vi "Actor Core.vi"(8 "error in":errorcluster, 11 "Rack Controller in":refnum<class "Rack Controller.lvclass">) -> (0 "error out":errorcluster, 3 "Actor out":refnum<class "Actor.lvclass">)   [LabVIEW 2019, in "Rack Controller.lvclass"]
doc: "(<B>Filename</B>: Actor Framework.lvlib:Actor.lvclass:Actor Core.vi)\n\nReceives messages to the actor, reacts to them, and initiates any error handling that may shut the actor down.\n\nDescendant classes may override this VI to append parallel tasks for the actor to complete while it handles messages. Overrides use the Call Parent Method node."
uses:
  Rack Controller.lvclass
  <vilib>/ActorFramework/Actor/Actor.lvclass
  <vilib>/ActorFramework/Stop Msg/Stop Msg.lvclass
  <vilib>/ActorFramework/Message Enqueuer/Message Enqueuer.lvclass
  Algorithm/FrameworkOverrides/Algorithm.lvclass
  <vilib>/vision/Image Controls.llb/IMAQ Image.ctl
  Controls/RC Local Data.ctl
  Controls/Output Cluster_RC.ctl
  Common/Controls/Camera Optics Diagnostics Result.ctl
  Common/Controls/Camera Optics Diagnostics.ctl
  Inspection Statemachine/Controls/Result Cluster_SM.ctl
  Inspection Statemachine/Inspection Statemachine.lvclass
  Controls/Part Details_RC.ctl
  Common/Controls/AllPartInfo.ctl
  <vilib>/event_ctls.llb/usereventprio.ctl
  ZenCAM/Camera Controller/Camera Controller Actor/Camera Controller.lvclass
  C:/Program Files/National Instruments/LabVIEW 2019/vi.lib/ActorFramework/Actor/Actor.lvclass
panel:
  out "Part Name":string
  out "RackId":i32
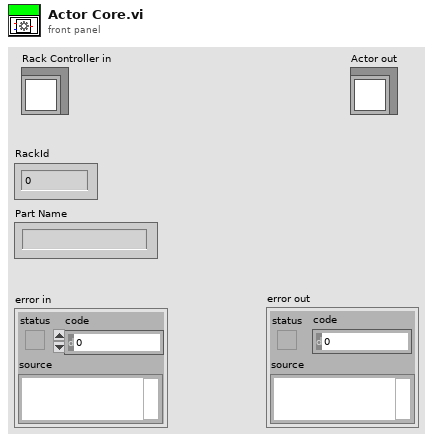
[diagram p1: front panel]
types:
  T1 = typedef "IMAQ Image.ctl" = refnum<image>
  T2 = cluster{"Buffer":cluster{"Result Cluster":cluster{"Rack ID":u8, "Measurement Values Array ":dbl[], "Images Array":T1[], "Result PF":bool, "Production Count Details":cluster{"Total Fail":u64, "Total Pass":u64, "Total Count":u64}, "Reel Count Details":cluster{"Reel Fail":u64, "Reel Pass":u64, "Reel Count":u64}, "Control PF Array":bool[], "Specification PF Array":bool[], "Specification Fail?":bool, "Reel Number":u64, "Status":string}, "Pause on Fail?":bool, "Total Count Finish?":bool, "Reel Count Finish?":bool}[], "Result Count":u32, "Swithch?":bool, "Check Pos 3":u32, "Global Count":u32, "Check Pos 1":u32, "Check Pos 2":u32, "Result ":cluster{"Result Cluster":cluster{"Rack ID":u8, "Measurement Values Array ":dbl[], "Images Array":T1[], "Result PF":bool, "Production Count Details":cluster{"Total Fail":u64, "Total Pass":u64, "Total Count":u64}, "Reel Count Details":cluster{"Reel Fail":u64, "Reel Pass":u64, "Reel Count":u64}, "Control PF Array":bool[], "Specification PF Array":bool[], "Specification Fail?":bool, "Reel Number":u64, "Status":string}, "Pause on Fail?":bool, "Total Count Finish?":bool, "Reel Count Finish?":bool}, "Image buffer":T1[][], "Buffer Size":u32}
  T3 = typedef "Rack Controller.lvclass/RC Local Data.ctl" = cluster{"Timeout":i32, "Core":cluster{"Current VI Reference":refnum<vi>, "Close Panel on Exit?":bool}, "Rack Id":u8, "Part Details":T4, "Ack":i32, "First Call?":bool, "Send Run to CC?":bool, "State":string, "Reel Number":u64, "Output Cluster":T5, "System Info_RC":cluster{"HardwareEmulated":bool, "DefectTrackingEnable":bool, "PauseOnReelCountFinish":bool, "StopOnTotalCountFinish":bool}, "Rack based Parameters":variant, "Update":bool, "CountDetails":cluster{"Total Cluster Values":cluster{"Total Fail":u64, "Total Pass":u64, "Total Count":u64}, "Reel Counter Cluster":cluster{"Reel Fail":u64, "Reel Pass":u64, "Reel Count":u64}}}
  T4 = typedef "Rack Controller.lvclass/Part Details_RC.ctl" = cluster{"Name":string, "Unload Position Counts":cluster{"Fail":u32, "Reel End":u32, "Production End":u32}, "Number Of Cameras":u8, "Measurement Details Array":cluster{"Measuement ID":u16, "Measurement Name":string, "Measurement Enable":bool, "CL Violation Threshold":cluster{"M":u8, "N":u64}, "SL Violation Threshold":cluster{"M":u8, "N":u64}, "CL Fail Count Array":u64[], "SL Fail Count Array":u64[]}[], "Reel Count":u64, "Total Count":u64}
  T5 = typedef "Rack Controller.lvclass/Output Cluster_RC.ctl" = cluster{"Acknowledgement":cluster{"Actor Enqueuer":refnum<class "Message Enqueuer.lvclass">, "VI Reference":refnum<vi>, "VI Name":string}, "Rack ID":u8, "Clear":bool, "Light Camera Info":T6, "Camera Optics Diagnostics Result":T7, "Receiver Enqueuer":cluster{"Actor Enqueuer":refnum<class "Message Enqueuer.lvclass">, "VI Name":string}, "Error Message":string, "Part Details":cluster{"Part Name":string, "Total Count":u64, "Reel Count":u64}, "Result Cluster":T8, "Part Info":cluster{"Part Name":string, "Rack ID":u8, "MeasurementIDsArray":u16[], "Measurement Names Array":string[], "Spec Values Array":cluster{"LCL":dbl, "UCL":dbl, "LSL":dbl, "USL":dbl, "Nominal Value":dbl}[], "Camera Names Array":string[], "Total count":u64, "Reel count":u64}, "AllPartInfo":T9, "ImagesAndCount":cluster{"Image Array":T1[], "ImageCount":u64}}
  T6 = typedef "Camera Optics Diagnostics.ctl" = cluster{"Light Camera Name":string, " State":string}
  T7 = typedef "Camera Optics Diagnostics Result.ctl" = cluster{"LightCameraName":string, "DiagnosedImage":T1, "DustPercentage":dbl, "Result":bool}
  T8 = typedef "Inspection Statemachine.lvclass/Result Cluster_SM.ctl" = cluster{"RackID":u8, "MeasurementValuesArray ":dbl[], "ImagesArray":T1[], "ResultPF":bool, "ProductionCountDetails":cluster{"TotalFail":u64, "TotalPass":u64, "TotalCount":u64}, "ReelCountDetails":cluster{"ReelFail":u64, "ReelPass":u64, "ReelCount":u64}, "ControlPFArray":bool[], "SpecificationPFArray":bool[], "SpecificationFail":bool, "ReelNumber":u64, "Status":string}
  T9 = typedef "AllPartInfo.ctl" = cluster{"PartName":string, "NumberOfRacks":u8, "MeasurementIDsArray":u16[], "MeasurementNamesArray":string[], "SpecValuesArray":cluster{"LCL":dbl, "UCL":dbl, "LSL":dbl, "USL":dbl, "NominalValue":dbl}[]}[]
  T10 = enum32{"invalid app kind", "Development System", "Run Time System", "Student Edition", "Embedded LabVIEW", "Evaluation", "Custom"}
  T11 = enum32{"Invalid", "Standard", "Closed", "Hidden", "Minimized", "Maximized"}
  T12 = cluster{"Unload Position Counts":cluster{"Fail":u32, "ReelEnd":u32, "ProductionEnd":u32}, "Number of Cameras":u8}
  T13 = cluster{"Reel Fail":u64, "Reel Pass":u64, "Reel Count":u64}
  T14 = cluster{"LCL":dbl, "UCL":dbl, "LSL":dbl, "USL":dbl, "NominalValue":dbl}[]
  T15 = cluster{"Total Cluster Values":cluster{"Total Fail":u64, "Total Pass":u64, "Total Count":u64}, "Reel Counter Cluster":cluster{"Reel Fail":u64, "Reel Pass":u64, "Reel Count":u64}}
  T16 = cluster{"Total Fail":u64, "Total Pass":u64, "Total Count":u64}
  T17 = cluster{"TotalFail":u64, "TotalPass":u64, "TotalCount":u64}
  T18 = cluster{"ReelFail":u64, "ReelPass":u64, "ReelCount":u64}
  T19 = cluster{"HardwareEmulated":bool, "DefectTrackingEnable":bool, "PauseOnReelCountFinish":bool, "StopOnTotalCountFinish":bool}
  T20 = cluster{"Current VI Reference":refnum<vi>, "Close Panel on Exit?":bool}
  T21 = cluster{"Fail":u32, "Reel End":u32, "Production End":u32}
  T22 = cluster{"Result Cluster":cluster{"Rack ID":u8, "Measurement Values Array ":dbl[], "Images Array":T1[], "Result PF":bool, "Production Count Details":cluster{"Total Fail":u64, "Total Pass":u64, "Total Count":u64}, "Reel Count Details":cluster{"Reel Fail":u64, "Reel Pass":u64, "Reel Count":u64}, "Control PF Array":bool[], "Specification PF Array":bool[], "Specification Fail?":bool, "Reel Number":u64, "Status":string}, "Pause on Fail?":bool, "Total Count Finish?":bool, "Reel Count Finish?":bool}
  T23 = cluster{"Measuement ID":u16, "Measurement Name":string, "Measurement Enable":bool, "CL Violation Threshold":cluster{"M":u8, "N":u64}, "SL Violation Threshold":cluster{"M":u8, "N":u64}, "CL Fail Count Array":u64[], "SL Fail Count Array":u64[]}[]
  T24 = typedef "usereventprio.ctl" = enum32{"high priority", "normal priority"}
  T25 = cluster{"Result Cluster":cluster{"Rack ID":u8, "Measurement Values Array ":dbl[], "Images Array":T1[], "Result PF":bool, "Production Count Details":cluster{"Total Fail":u64, "Total Pass":u64, "Total Count":u64}, "Reel Count Details":cluster{"Reel Fail":u64, "Reel Pass":u64, "Reel Count":u64}, "Control PF Array":bool[], "Specification PF Array":bool[], "Specification Fail?":bool, "Reel Number":u64, "Status":string}, "Pause on Fail?":bool, "Total Count Finish?":bool, "Reel Count Finish?":bool}[]
  T26 = cluster{"Rack ID":u8, "Measurement Values Array ":dbl[], "Images Array":T1[], "Result PF":bool, "Production Count Details":cluster{"Total Fail":u64, "Total Pass":u64, "Total Count":u64}, "Reel Count Details":cluster{"Reel Fail":u64, "Reel Pass":u64, "Reel Count":u64}, "Control PF Array":bool[], "Specification PF Array":bool[], "Specification Fail?":bool, "Reel Number":u64, "Status":string}
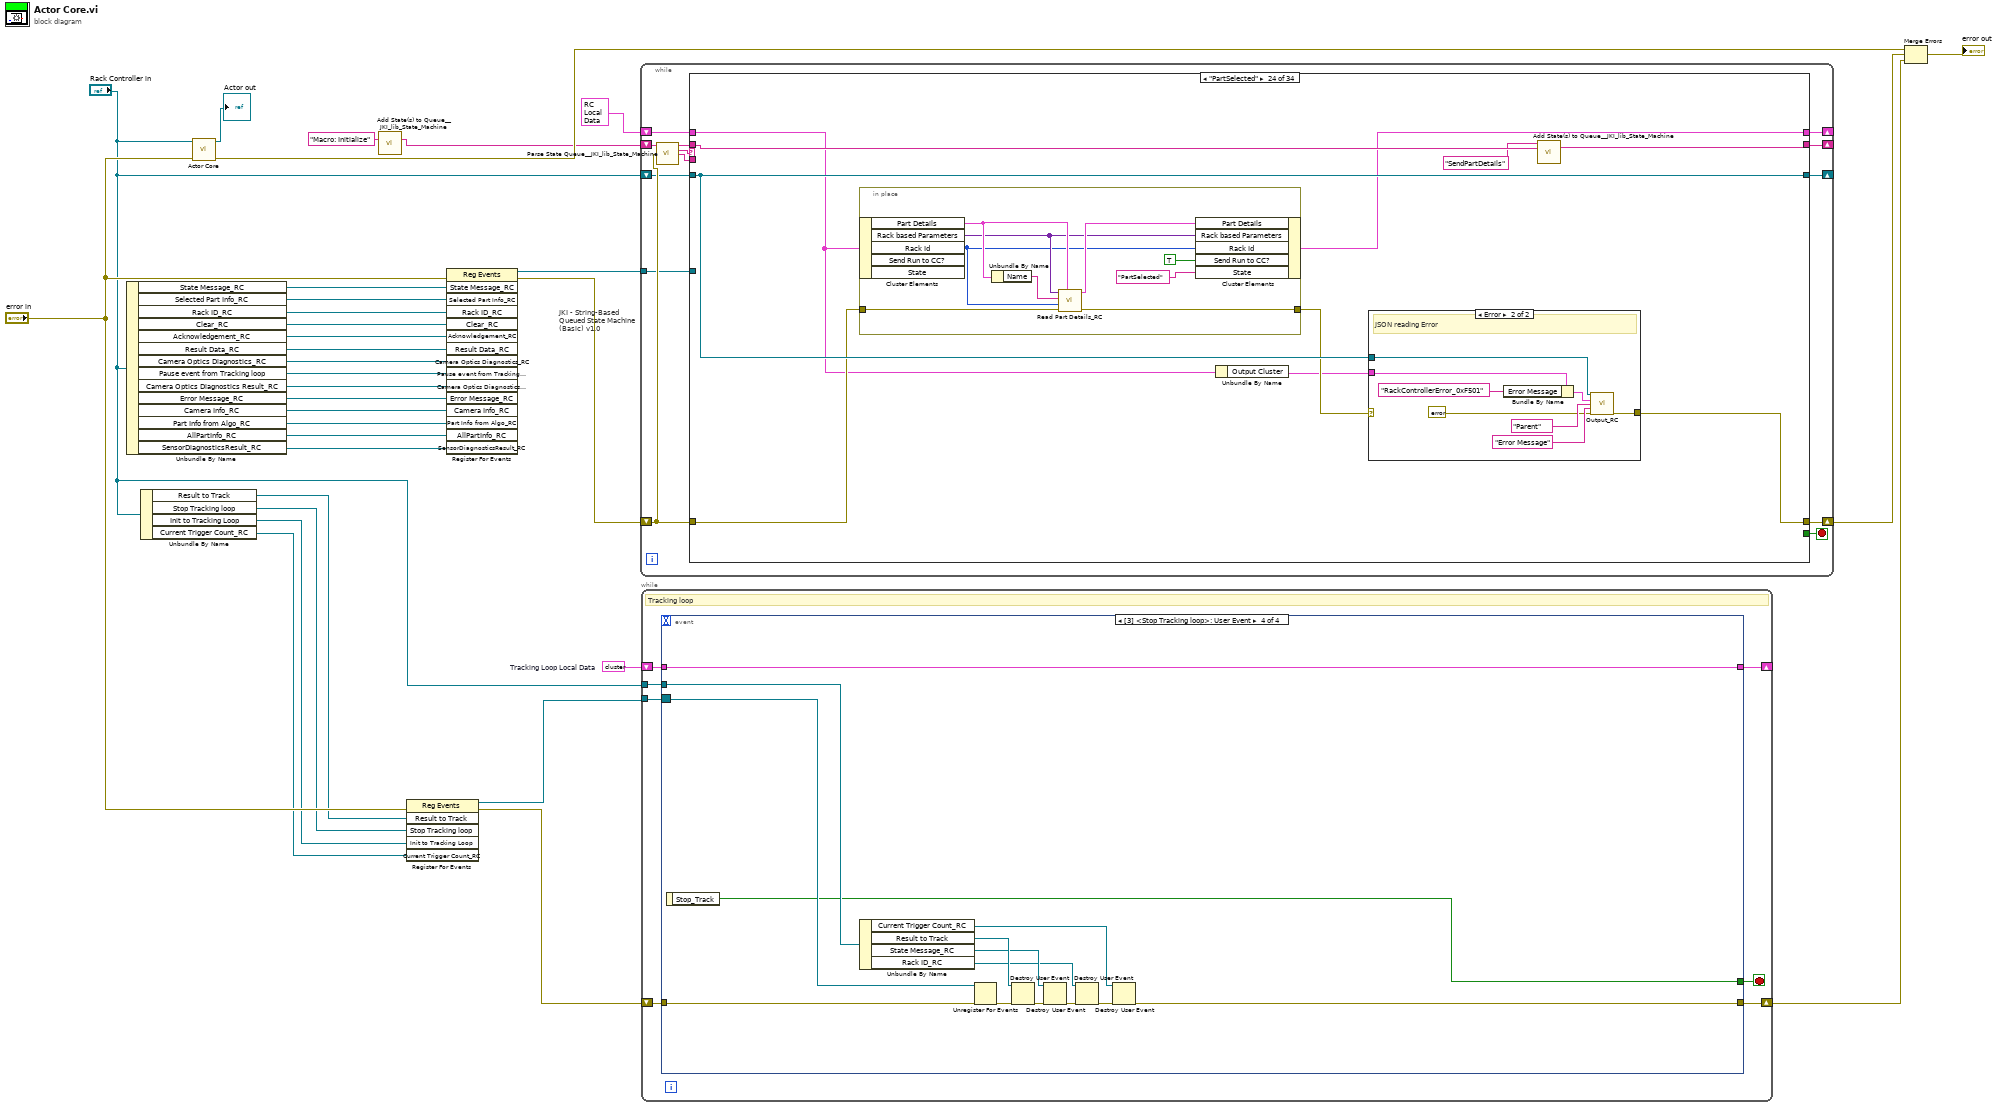
[diagram p0: block diagram]
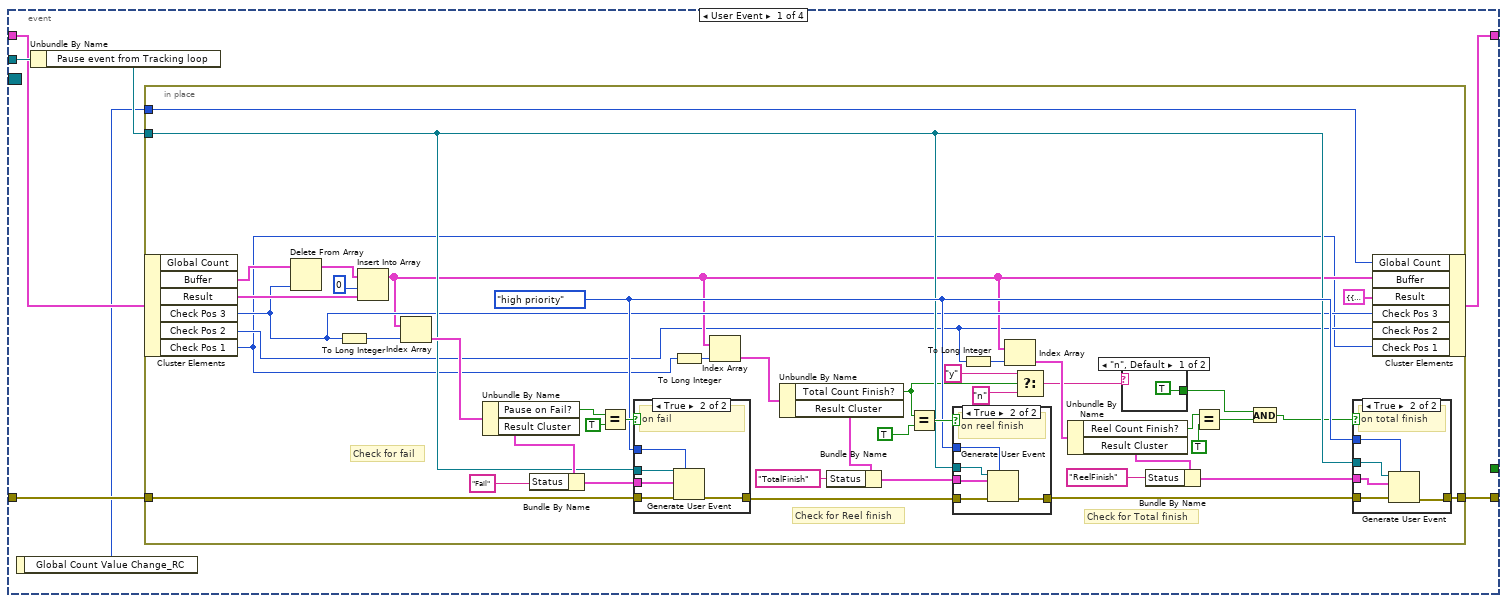
[diagram p2: hidden frame]
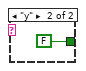
[diagram p3: hidden frame]
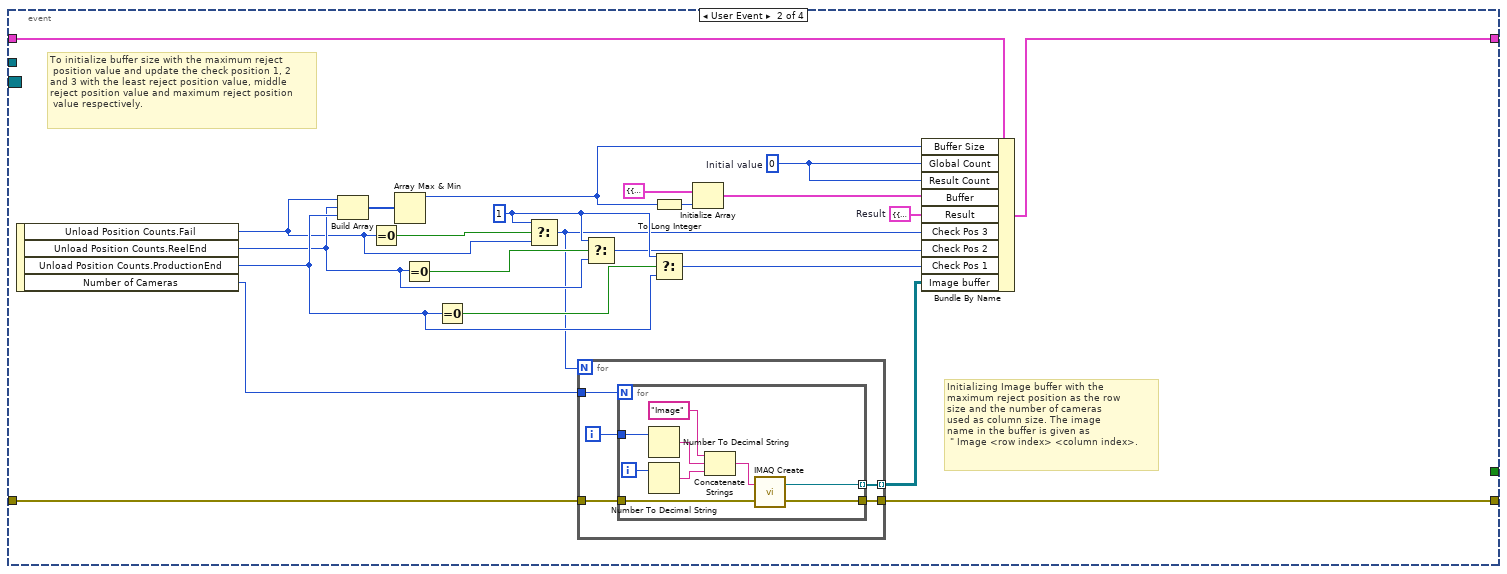
[diagram p7: hidden frame]
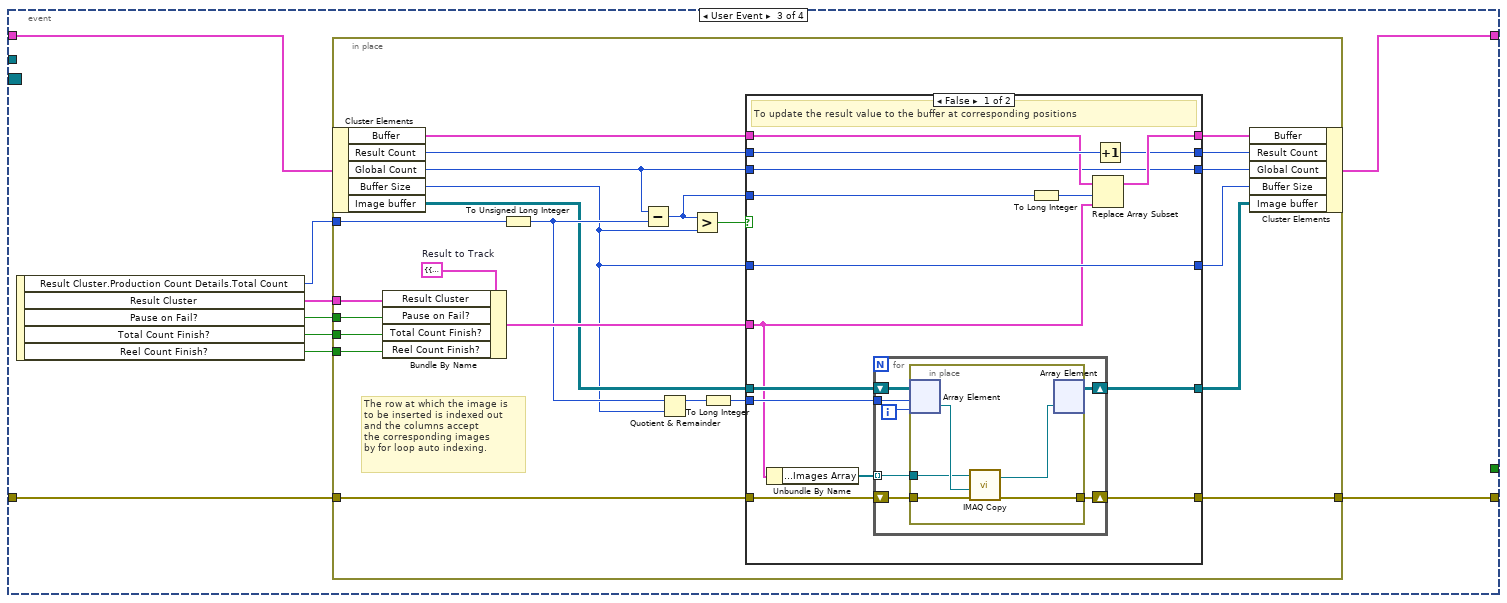
[diagram p8: hidden frame]
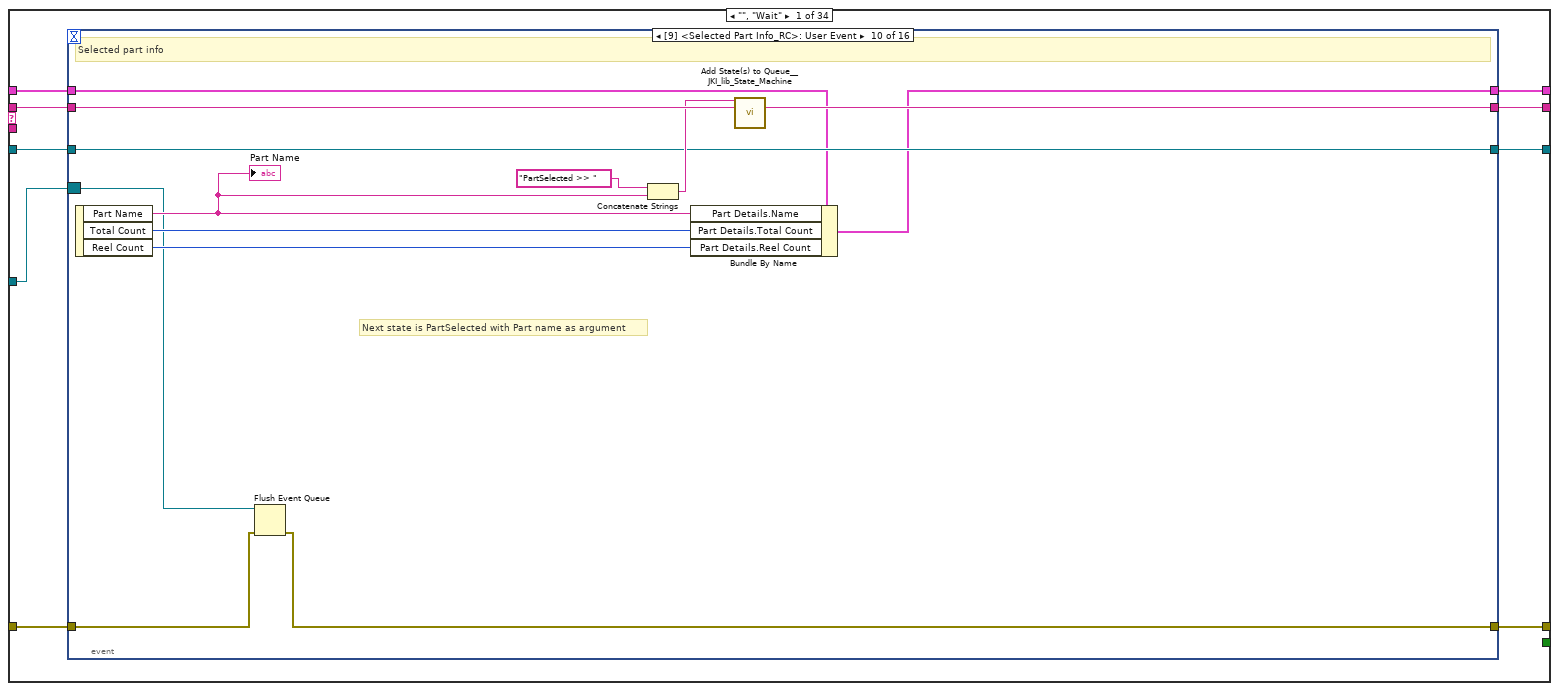
[diagram p10: hidden frame]
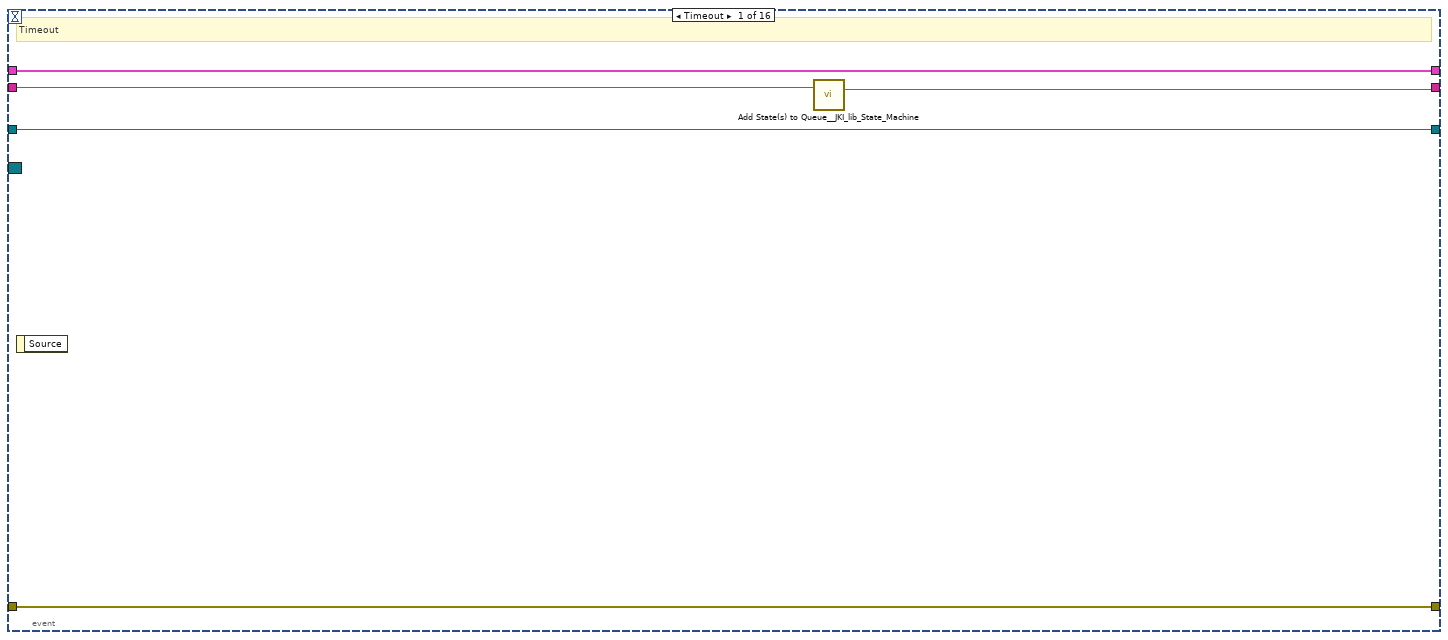
[diagram p11: hidden frame]
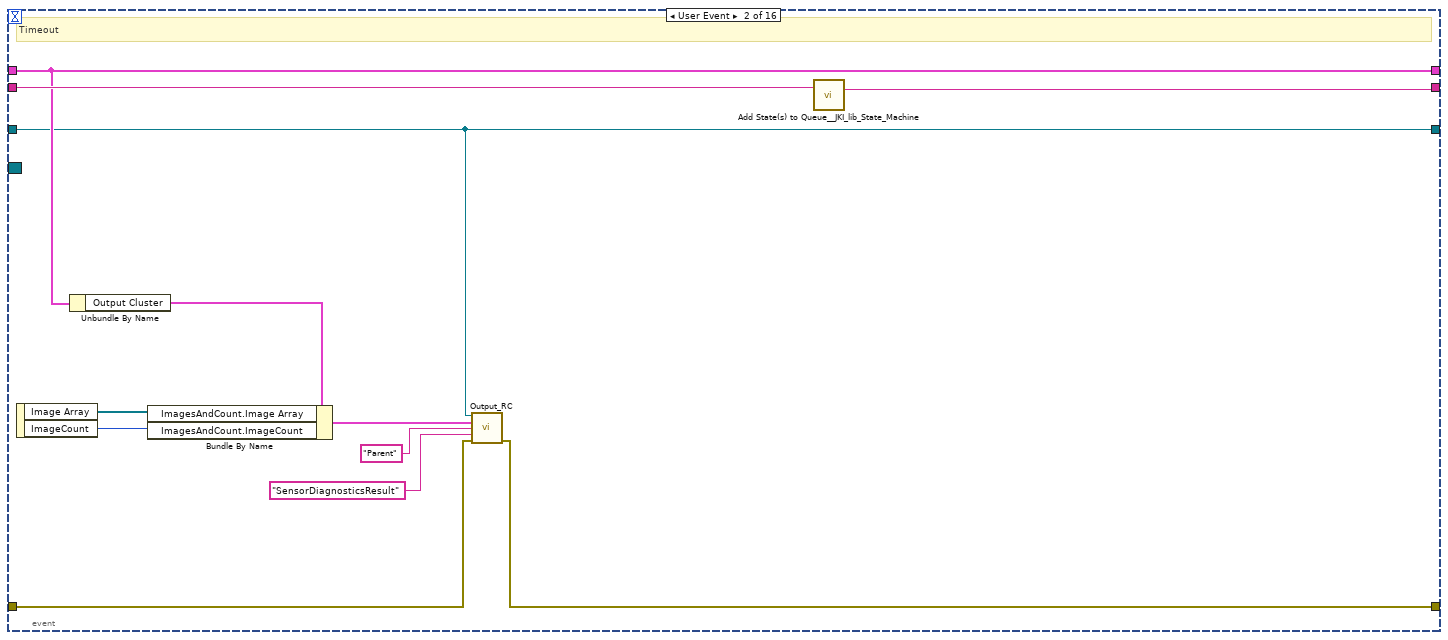
[diagram p12: hidden frame]
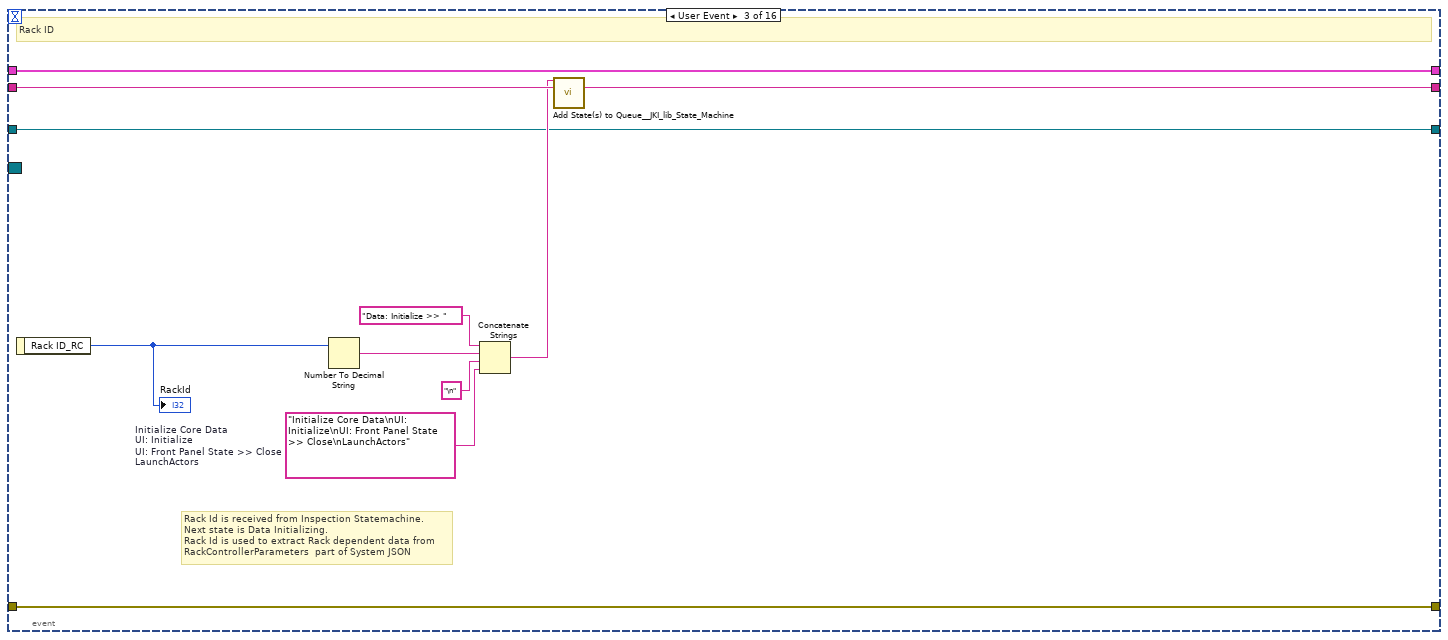
[diagram p13: hidden frame]
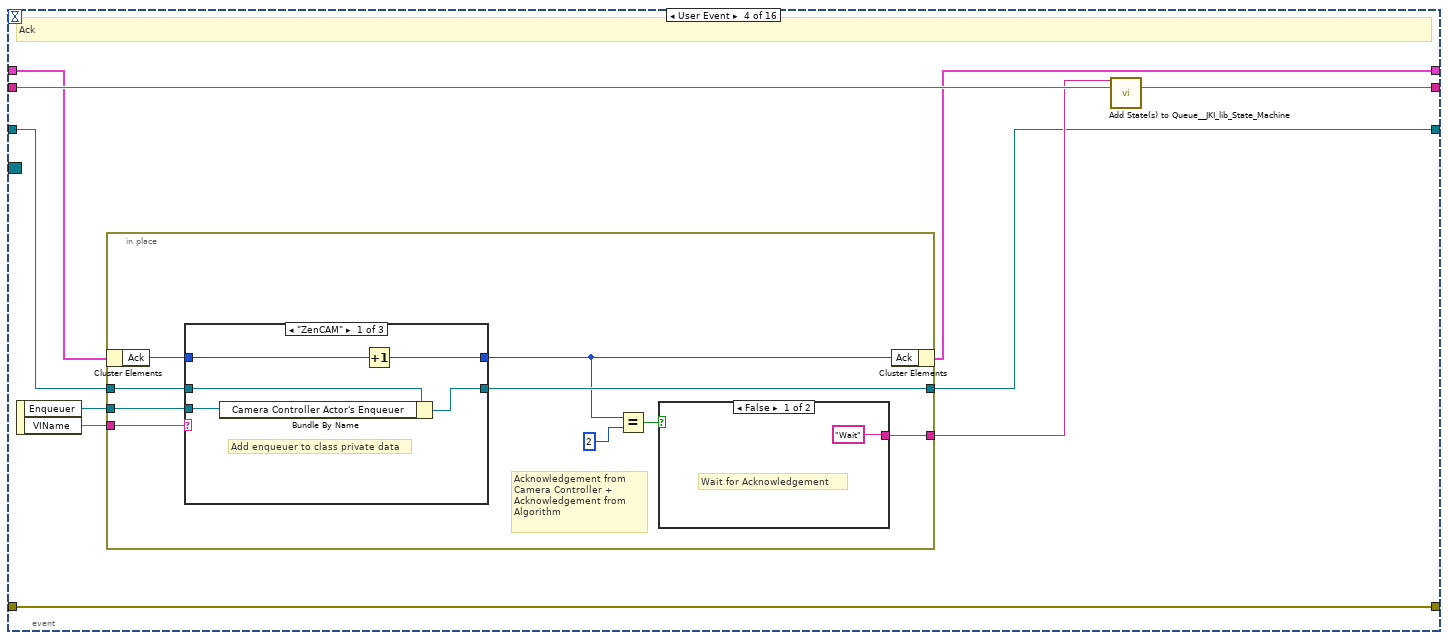
[diagram p14: hidden frame]
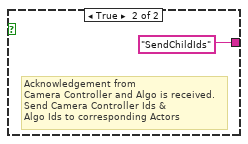
[diagram p15: hidden frame]
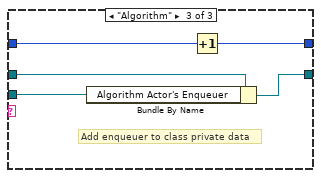
[diagram p17: hidden frame]
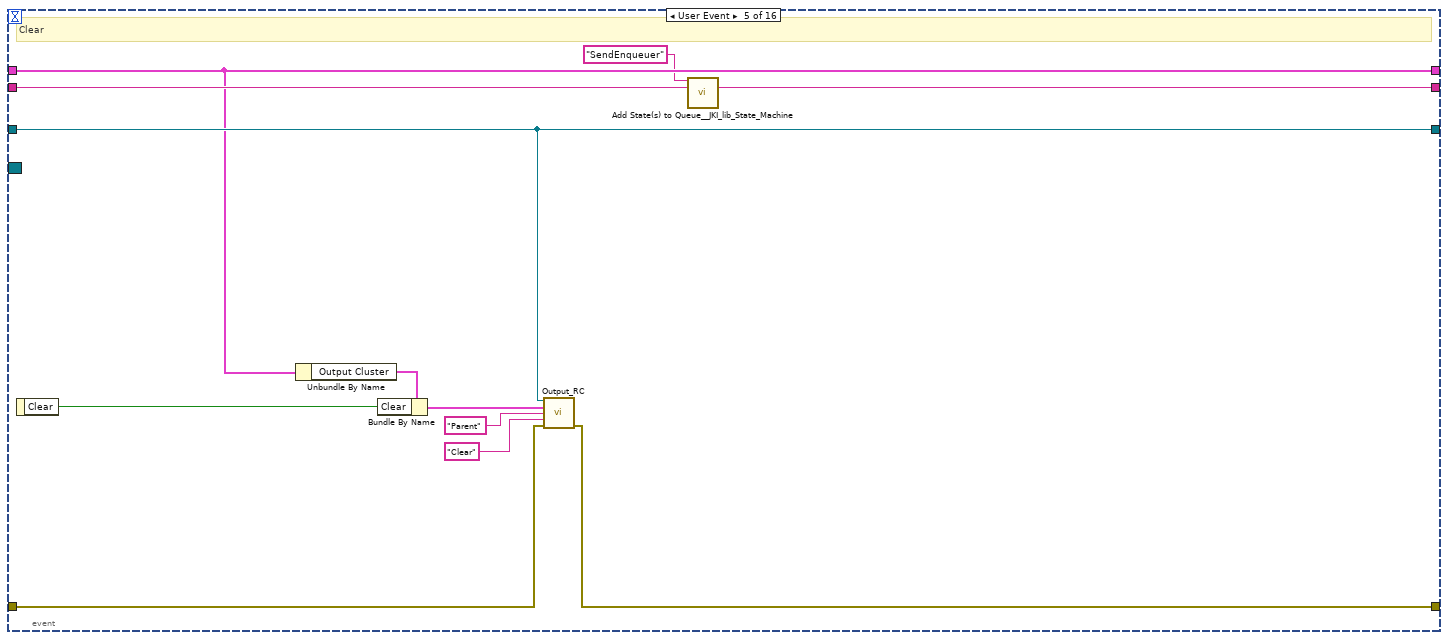
[diagram p18: hidden frame]
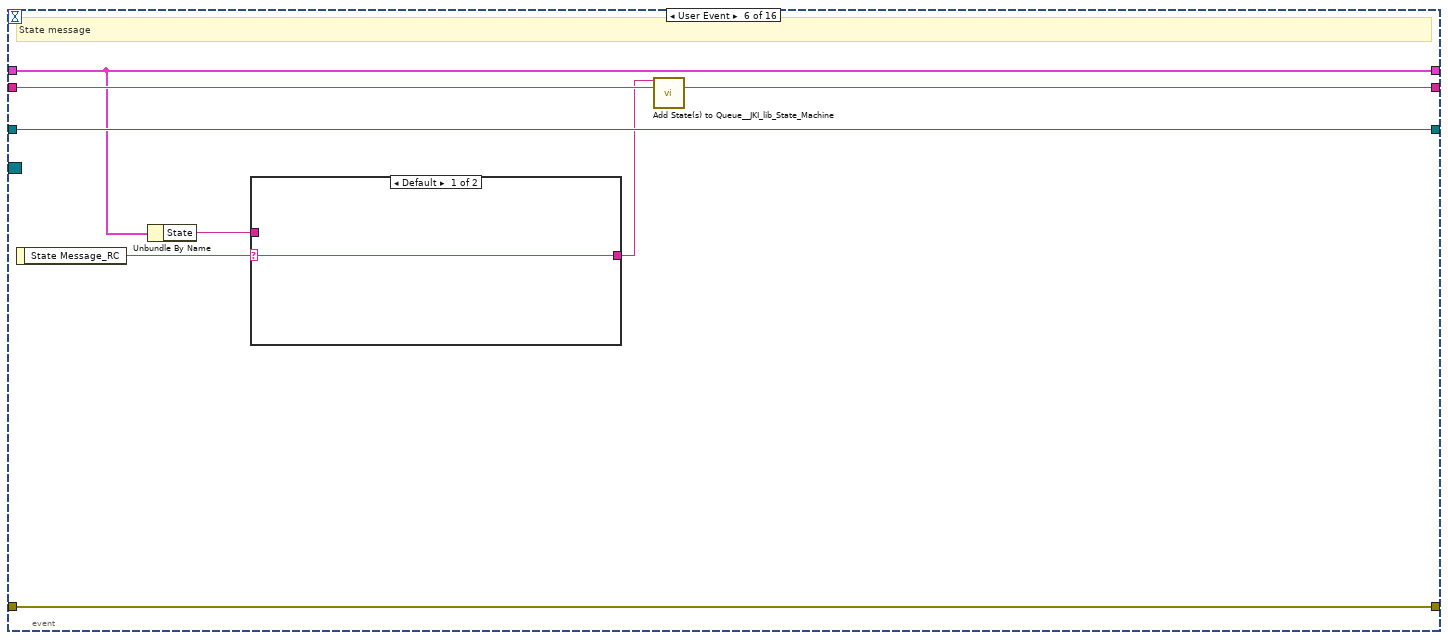
[diagram p19: hidden frame]
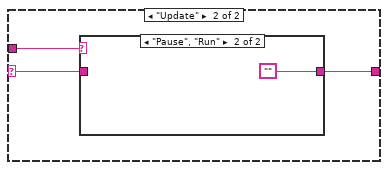
[diagram p20: hidden frame]
diagram:
  w7 = T2 {"Buffer"=[{"Result Cluster"={"Rack ID"=0, "Measurement Values Array "=[], "Images Array"=[], "Result PF"=TRUE, "Production Count Details"={"Total Fail"=0, "Total Pass"=0, "Total Count"=0}, "Reel Count Details"={"Reel Fail"=0, "Reel Pass"=0, "Reel Count"=0}, "Control PF Array"=[], "Specification PF Array"=[], "Specification Fail?"=FALSE, "Reel Number"=0, "Status"=""}, "Pause on Fail?"=FALSE, "Total Count Finish?"=FALSE, "Reel Count Finish?"=FALSE}], "Result Count"=0, "Swithch?"=FALSE, "Check Pos 3"=0, "Global Count"=0, "Check Pos 1"=0, "Check Pos 2"=0, "Result "={"Result Cluster"={"Rack ID"=0, "Measurement Values Array "=[], "Images Array"=[], "Result PF"=TRUE, "Production Count Details"={"Total Fail"=0, "Total Pass"=0, "Total Count"=0}, "Reel Count Details"={"Reel Fail"=0, "Reel Pass"=0, "Reel Count"=0}, "Control PF Array"=[], "Specification PF Array"=[], "Specification Fail?"=FALSE, "Reel Number"=0, "Status"=""}, "Pause on Fail?"=FALSE, "Total Count Finish?"=FALSE, "Reel Count Finish?"=FALSE}, "Image buffer"=[], "Buffer Size"=0}  # Tracking Loop Local Data
  n1 = Unbundle By Name("Rack Controller in") -> ("State Message_RC"=w17:refnum<user-event>, "Selected Part Info_RC"=w27:refnum<user-event>, "Rack ID_RC"=w26:refnum<user-event>, "Clear_RC"=w25:refnum<user-event>, "Acknowledgement_RC"=w24:refnum<user-event>, "Result Data_RC"=w23:refnum<user-event>, "Camera Optics Diagnostics_RC"=w22:refnum<user-event>, "Pause event from Tracking loop"=w21:refnum<user-event>, "Camera Optics Diagnostics Result_RC"=w20:refnum<user-event>, "Error Message_RC"=w19:refnum<user-event>, "Camera Info_RC"=w14:refnum<user-event>, "Part Info from Algo_RC"=w9:refnum<user-event>, "AllPartInfo_RC"=w2:refnum<user-event>, "SensorDiagnosticsResult_RC"=w1:refnum<user-event>)
  n2 = Unbundle By Name("Rack Controller in") -> ("Result to Track"=w10:refnum<user-event>, "Stop Tracking loop"=w11:refnum<user-event>, "Init to Tracking Loop"=w12:refnum<user-event>, "Current Trigger Count_RC"=w13:refnum<user-event>)
  n3 = call-parent "Actor Core.vi"("error in"="error in", "Actor in"="Rack Controller in") -> ("error out"=w31:errorcluster, "Actor out"=→"Actor out":refnum<class "Actor.lvclass">)  [unwired: 8 in]
  n4 = call <vilib>:"Add State(s) to Queue__JKI_lib_State_Machine.vi"("State(s) in (\"\")"="Macro: Initialize") -> ("States Out"=w18:string)  [unwired: 14 in]
  n5 = register-events(error in="error in", w10, w11, w12, w13) -> (reference out=w6:refnum<event-registration>, error out=w4:errorcluster)  [unwired: 1 in]
  n6 = register-events(error in="error in", w17, w27, w26, w25, w24, w23, w22, w21, w20, w19, w14, w9, w2, w1) -> (reference out=w29:refnum<event-registration>, error out=w16:errorcluster)  [unwired: 1 in]
  n7 = while "JKI - String-Based Queued State Machine (Basic) v1.0" {
    shift-right: [w41] -> _
    shift-left: T3 {"Timeout"=0, "Core"={"Current VI Reference"=refnum, "Close Panel on Exit?"=FALSE}, "Rack Id"=0, "Part Details"={"Name"="", "Unload Position Counts"={"Fail"=0, "Reel End"=0, "Production End"=0}, "Number Of Cameras"=0, "Measurement Details Array"=[], "Reel Count"=0, "Total Count"=0}, "Ack"=0, "First Call?"=FALSE, "Send Run to CC?"=FALSE, "State"="", "Reel Number"=0, "Output Cluster"={"Acknowledgement"={"Actor Enqueuer"=refnum, "VI Reference"=refnum, "VI Name"=""}, "Rack ID"=0, "Clear"=FALSE, "Light Camera Info"={"Light Camera Name"="", " State"=""}, "Camera Optics Diagnostics Result"={"LightCameraName"="", "DiagnosedImage"=refnum, "DustPercentage"=0.0, "Result"=TRUE}, "Receiver Enqueuer"={"Actor Enqueuer"=refnum, "VI Name"=""}, "Error Message"="", "Part Details"={"Part Name"="", "Total Count"=0, "Reel Count"=0}, "Result Cluster"={"RackID"=0, "MeasurementValuesArray "=[], "ImagesArray"=[], "ResultPF"=FALSE, "ProductionCountDetails"={"TotalFail"=0, "TotalPass"=0, "TotalCount"=0}, "ReelCountDetails"={"ReelFail"=0, "ReelPass"=0, "ReelCount"=0}, "ControlPFArray"=[], "SpecificationPFArray"=[], "SpecificationFail"=FALSE, "ReelNumber"=0, "Status"=""}, "Part Info"={"Part Name"="", "Rack ID"=0, "MeasurementIDsArray"=[], "Measurement Names Array"=[], "Spec Values Array"=[], "Camera Names Array"=[], "Total count"=0, "Reel count"=0}, "AllPartInfo"=[{"PartName"="", "NumberOfRacks"=0, "MeasurementIDsArray"=[], "MeasurementNamesArray"=[], "SpecValuesArray"=[]}], "ImagesAndCount"={"Image Array"=[], "ImageCount"=0}}, "System Info_RC"={"HardwareEmulated"=TRUE, "DefectTrackingEnable"=TRUE, "PauseOnReelCountFinish"=TRUE, "StopOnTotalCountFinish"=TRUE}, "Rack based Parameters"=variant, "Update"=FALSE, "CountDetails"={"Total Cluster Values"={"Total Fail"=0, "Total Pass"=0, "Total Count"=0}, "Reel Counter Cluster"={"Reel Fail"=0, "Reel Pass"=0, "Reel Count"=0}}} ("cluster") -> [w40]
    shift-right: [w35] -> w28
    shift-left: w16 -> [w39]
    shift-right: [w42] -> _
    shift-left: w18 -> [w43]
    tunnel: w29 -> [w37]
    shift-right: [w36] -> _
    shift-left: "Rack Controller in" -> [w38]
    stop <- w34 stop-if-true
    n8 = call <vilib>:"Parse State Queue__JKI_lib_State_Machine.vi"("State Queue"=w43, "Error In (no error)"=w39) -> ("Remaining States"=w45:string, "Current State"=w46:string, "Arguments"=w44:string)  [unwired: 11 in]
    n9 = case shown="\"PartSelected\"" w46 {
      selector: w46 -> [_ _ w322 _ _ _ _ _ _ _ _ _ _ _ _ _ _ _ _ _ _ _ _ _ _ _ _ _ _ _ _ _ _ _]
      tunnel: w45 -> [w55 w318 w324 w343 w354 w360 w365 w391 w401 w406 w411 w419 w446 w452 w464 w469 w484 w494 w508 w518 w525 w534 w543 w553 w587 w609 w629 w639 w687 w707 w802 w812 w822 w835]
      tunnel: w44 -> [_ _ _ _ _ _ _ w386 _ _ _ w412 _ _ _ _ _ _ _ _ _ _ _ _ _ _ _ _ _ _ _ _ _ _]
      tunnel: w40 -> [w53 w315 w320 w334 w349 w358 w362 _ w398 w403 w409 w415 w443 w450 w461 w466 w473 w492 w506 w515 w522 w530 w538 w545 w585 w606 w624 w632 w666 w692 w789 w807 w817 w833]
      tunnel: [w52 w316 w326 w340 errorcluster {"status"=FALSE, "code"=0, "source"=""} ("error out") w357 w363 w372 w399 w404 w408 w416 w444 w447 w462 w467 w481 w488 w495 w516 w523 w531 w539 w551 w577 w591 w625 w635 w681 w700 w795 w808 w818 w823] -> w35
      tunnel: w39 -> [w51 w316 w325 w340 _ w357 w363 w373 w396 w404 w408 w417 w444 w447 w462 w467 w482 w490 w505 w517 w523 w532 w540 w548 w578 w600 w626 w637 w669 w704 w787 w803 w813 w824]
      tunnel: [w54 w317 w323 w342 w353 w359 w364 w390 w400 w405 w410 w418 w445 w451 w463 w468 w483 w493 w507 w519 w524 w533 w542 w552 w586 w608 w628 w638 w686 w706 w801 w811 w821 w834] -> w42
      tunnel: [_ _ _ _ _ TRUE _ _ _ _ _ _ _ _ TRUE _ _ _ _ _ _ _ _ _ _ _ _ _ _ _ _ _ _ _] -> w34
      tunnel: [w49 w315 w320 w341 w349 w358 w362 w383 w398 w403 w409 w415 w443 w450 w461 w466 w472 w492 w506 w515 w522 w530 w538 w546 w585 w607 w624 w631 w670 w694 w799 w807 w817 w833] -> w41
      tunnel: w38 -> [w48 w314 w321 w332 w350 w355 w361 w376 w393 w402 w407 w414 w442 w448 w457 w465 w480 w487 w498 w512 w520 w529 w541 w550 w584 w599 w623 w634 w682 w689 w790 w809 w819 w825]
      tunnel: w37 -> [w50 _ _ _ _ _ _ _ w397 _ _ _ _ _ _ _ _ _ _ _ _ _ _ _ _ _ _ _ _ w698 w798 _ _ _]
      tunnel: [w47 w314 w321 w332 w350 w355 w361 w376 w393 w402 w407 w414 w442 w448 w457 w465 w480 w487 w498 w512 w520 w529 w541 w550 w584 w599 w623 w634 w682 w689 w790 w809 w819 w825] -> w36
      frame "", "Wait" {
        n10 = event shown="[9] <Selected Part Info_RC>: User Event" {
          selector: w50 -> [_ _ _ _ _ _ _ _ _ w180 _ _ _ _ _ _]
          dyn-events: _ -> [_ _ _ _ _ _ _ _ _ _ _ _ _ _ _ _]
          timeout: _ -> [_ _ _ _ _ _ _ _ _ _ _ _ _ _ _ _]
          tunnel: w55 -> [w60 w72 w82 w92 w127 w136 w153 w165 w179 w192 w210 w223 w232 w261 w294 w313]
          tunnel: [w59 w71 w81 w93 w128 w135 w152 w164 w178 w188 w209 w222 w231 w262 w295 w312] -> w54
          tunnel: w53 -> [w58 w69 w83 w85 w125 w130 w151 w163 w177 w187 w204 w221 w228 w240 w286 w310]
          tunnel: [w56 w62 w80 w86 w121 w133 w148 w154 w172 w181 w200 w214 w229 w255 w292 w311] -> w52
          tunnel: w51 -> [w56 w63 w80 w86 w120 w133 w143 w155 w173 w182 w199 w215 w229 w247 w293 w311]
          tunnel: [w58 w69 w83 w84 w125 w130 w151 w163 w177 w186 w203 w221 w227 w250 w286 w310] -> w49
          tunnel: w48 -> [w57 w65 w76 w91 w126 w134 w147 w159 w176 w189 w208 w220 w230 w254 w291 w307]
          tunnel: [w57 w65 w76 w89 w126 w134 w147 w159 w176 w189 w208 w220 w230 w254 w291 w307] -> w47
          event Timeout {
            # "Timeout"
            n11 = event-data() -> ()  [unwired: 1 in, 1 out]
            n12 = call <vilib>:"Add State(s) to Queue__JKI_lib_State_Machine.vi"("State(s) in (\"\")"=w60) -> ("States Out"=w59:string)  [unwired: 14 in]
          }
          event User Event {
            # "Timeout"
            n13 = event-data() -> ("Image Array"=w67:T1[], "ImageCount"=w66:u64)  [unwired: 1 in]
            n14 = Unbundle By Name(w69) -> ("Output Cluster"=w68:T5)
            n15 = Bundle By Name(cluster=w68, "ImagesAndCount.Image Array"=w67, "ImagesAndCount.ImageCount"=w66) -> (w64:T5)
            n16 = call "Output_RC.vi"("Rack Controller in"=w65, "Output Cluster"=w64, "Receiver Name"="Parent", "State"="SensorDiagnosticsResult", "error in (no error)"=w63) -> ("error out"=w62:errorcluster)  [unwired: 10 in]
            n17 = call <vilib>:"Add State(s) to Queue__JKI_lib_State_Machine.vi"("State(s) in (\"\")"=w72) -> ("States Out"=w71:string)  [unwired: 14 in]
          }
          event User Event {
            w75 = "Initialize Core Data\nUI: Initialize\nUI: Front Panel State >> Close\nLaunchActors"  # Initialize Core Data UI: Initialize UI: Front Panel State >> Close LaunchActors
            # "Rack Id is received from Inspection Statemachine.\nNext state is Data Initializing.\nRack Id is used to extract Rack dependent data from\nRackControllerParameters  part of System JSON"
            # "Rack ID"
            n18 = event-data() -> ("Rack ID_RC"=w73:i32)  [unwired: 1 in]
            "RackId" <- w73
            n19 = Number To Decimal String(number=w73) -> (decimal integer string=w78:string)  [unwired: 1 in]
            n20 = Concatenate Strings("Data: Initialize >> ", w78, "\n" ("string"), w75) -> (w77:string)
            n21 = call <vilib>:"Add State(s) to Queue__JKI_lib_State_Machine.vi"("State(s) in Front (\"\")"=w77, "State(s) in (\"\")"=w82) -> ("States Out"=w81:string)  [unwired: 13 in]
          }
          event User Event {
            # "Ack"
            n22 = event-data() -> ("Enqueuer"=w88:refnum<class "Message Enqueuer.lvclass">, "VIName"=w87:string)  [unwired: 1 in]
            n23 = in-place {
              in-place-border: w91 -> [w102]
              in-place-border: [w101] -> w90
              in-place-border: [w98] -> w89
              in-place-border: w88 -> [w97]
              in-place-border: w87 -> [w96]
              # "Acknowledgement from\nCamera Controller +\nAcknowledgement from \nAlgorithm"
              n24 = in-place-cluster #1(w85) -> ("Ack"=w95:i32)
              n25 = case shown="\"ZenCAM\"" w96 {
                tunnel: w97 -> [w105 _ w112]
                tunnel: w102 -> [w107 w111 w114]
                tunnel: [w106 w111 w113] -> w98
                tunnel: w95 -> [w109 w110 w116]
                tunnel: [w108 w110 w115] -> w94
                frame "ZenCAM" {
                  # "Add enqueuer to class private data"
                  n26 = Bundle By Name(cluster=w107, "Camera Controller Actor's Enqueuer"=w105) -> (w106:refnum<class "Rack Controller.lvclass">)
                  n27 = Increment(x=w109) -> (x+1=w108:i32)
                }
                frame Default {
                }
                frame "Algorithm" {
                  # "Add enqueuer to class private data"
                  n28 = Bundle By Name(cluster=w114, "Algorithm Actor's Enqueuer"=w112) -> (w113:refnum<class "Rack Controller.lvclass">)
                  n29 = Increment(x=w116) -> (x+1=w115:i32)
                }
              }
              n30 = Equal?(x=w94, y=2) -> (x = y?=w100:bool)
              n31 = case shown="False" w100 {
                tunnel: ["Wait" ("State(s) in Front (\"\")") "SendChildIds" ("State(s) in Front (\"\")")] -> w101
                frame False {
                  # "Wait for Acknowledgement"
                }
                frame True {
                  # "Acknowledgement from \nCamera Controller and Algo is received.\nSend Camera Controller Ids & \nAlgo Ids to corresponding Actors"
                }
              }
              n32 = in-place-cluster #1("Ack"=w94) -> (w84:T3)
            }
            n33 = call <vilib>:"Add State(s) to Queue__JKI_lib_State_Machine.vi"("State(s) in Front (\"\")"=w90, "State(s) in (\"\")"=w92) -> ("States Out"=w93:string)  [unwired: 13 in]
          }
          event User Event {
            # "Clear"
            n34 = event-data() -> ("Clear"=w118:bool)  [unwired: 1 in]
            n35 = Unbundle By Name(w125) -> ("Output Cluster"=w124:T5)
            n36 = Bundle By Name(cluster=w124, "Clear"=w118) -> (w123:T5)
            n37 = call "Output_RC.vi"("Rack Controller in"=w126, "Output Cluster"=w123, "Receiver Name"="Parent", "State"="Clear", "error in (no error)"=w120) -> ("error out"=w121:errorcluster)  [unwired: 10 in]
            n38 = call <vilib>:"Add State(s) to Queue__JKI_lib_State_Machine.vi"("State(s) in Front (\"\")"="SendEnqueuer" ("State(s) in Front (\"\")"), "State(s) in (\"\")"=w127) -> ("States Out"=w128:string)  [unwired: 13 in]
          }
          event User Event {
            # "State message"
            n39 = event-data() -> ("State Message_RC"=w132:string)  [unwired: 1 in]
            n40 = Unbundle By Name(w130) -> ("State"=w129:string)
            n41 = case shown="Default" w132 {
              selector: w132 -> [w137 w138]
              tunnel: [w137 w139] -> w131
              tunnel: w129 -> [_ w140]
              frame Default {
              }
              frame "Update" {
                n42 = case shown="\"Pause\", \"Run\"" w140 {
                  tunnel: [w141 ""] -> w139
                  tunnel: w138 -> [w141 _]
                  frame Default {
                  }
                  frame "Pause", "Run" {
                  }
                }
              }
            }
            n43 = call <vilib>:"Add State(s) to Queue__JKI_lib_State_Machine.vi"("State(s) in Front (\"\")"=w131, "State(s) in (\"\")"=w136) -> ("States Out"=w135:string)  [unwired: 13 in]
          }
          event User Event {
            # "Error message"
            n44 = event-data() -> ("Error Message_RC"=w145:string)  [unwired: 1 in]
            n45 = Unbundle By Name(w151) -> ("Output Cluster"=w146:T5)
            n46 = Bundle By Name(cluster=w146, "Error Message"=w145) -> (w144:T5)
            n47 = call "Output_RC.vi"("Rack Controller in"=w147, "Output Cluster"=w144, "Receiver Name"="Parent", "State"="Error Message", "error in (no error)"=w143) -> ("error out"=w148:errorcluster)  [unwired: 10 in]
            n48 = call <vilib>:"Add State(s) to Queue__JKI_lib_State_Machine.vi"("State(s) in (\"\")"=w153) -> ("States Out"=w152:string)  [unwired: 14 in]
          }
          event User Event {
            # "Cam optics diagnostics"
            n49 = event-data() -> ("Light Camera Name"=w161:string, "State"=w160:string)  [unwired: 1 in]
            n50 = Unbundle By Name(w163) -> ("Output Cluster"=w162:T5)
            n51 = Bundle By Name(cluster=w162, "Light Camera Info.Light Camera Name"=w161, "Light Camera Info.State"=w160) -> (w158:T5)
            n52 = call "Output_RC.vi"("Rack Controller in"=w159, "Output Cluster"=w158, "Receiver Name"="ZenCAM", "State"="Camera Optics Diagnostics", "error in (no error)"=w155) -> ("error out"=w154:errorcluster)  [unwired: 10 in]
            n53 = call <vilib>:"Add State(s) to Queue__JKI_lib_State_Machine.vi"("State(s) in (\"\")"=w165) -> ("States Out"=w164:string)  [unwired: 14 in]
          }
          event User Event {
            # "Cam optics diagnostics result"
            n54 = event-data() -> ("Light Camera Name"=w170:string, "Diagnosed Image"=w169:T1, "Dust Percentage"=w168:dbl, "Result"=w167:bool)  [unwired: 1 in]
            n55 = Unbundle By Name(w177) -> ("Output Cluster"=w171:T5)
            n56 = Bundle By Name(cluster=w171, "Camera Optics Diagnostics Result.LightCameraName"=w170, "Camera Optics Diagnostics Result.DiagnosedImage"=w169, "Camera Optics Diagnostics Result.DustPercentage"=w168, "Camera Optics Diagnostics Result.Result"=w167) -> (w166:T5)
            n57 = call "Output_RC.vi"("Rack Controller in"=w176, "Output Cluster"=w166, "Receiver Name"="Parent", "State"="Camera Optics Diagnostics Result", "error in (no error)"=w173) -> ("error out"=w172:errorcluster)  [unwired: 10 in]
            n58 = call <vilib>:"Add State(s) to Queue__JKI_lib_State_Machine.vi"("State(s) in (\"\")"=w179) -> ("States Out"=w178:string)  [unwired: 14 in]
          }
          event User Event {
            # "Next state is PartSelected with Part name as argument"
            # "Selected part info"
            n59 = event-data() -> ("Part Name"=w183:string, "Total Count"=w184:u64, "Reel Count"=w185:u64)  [unwired: 1 in]
            "Part Name" <- w183
            n60 = Flush Event Queue(0:w180, 3:w182) -> (11:w181:errorcluster)  [unwired: 4 in, 2 out]
            n61 = Concatenate Strings("PartSelected >> " ("State(s) in Front (\"\")"), w183) -> (w190:string)
            n62 = Bundle By Name(cluster=w187, "Part Details.Name"=w183, "Part Details.Total Count"=w184, "Part Details.Reel Count"=w185) -> (w186:T3)
            n63 = call <vilib>:"Add State(s) to Queue__JKI_lib_State_Machine.vi"("State(s) in Front (\"\")"=w190, "State(s) in (\"\")"=w192) -> ("States Out"=w188:string)  [unwired: 13 in]
          }
          event User Event {
            # "Part info from algo"
            n64 = event-data() -> ("PartName"=w198:string, "MeasurementIDsArray"=w206:u16[], "MeasurementNamesArray"=w205:string[], "SpecValuesArray"=w201:T14)  [unwired: 1 in]
            n65 = Unbundle By Name(w204) -> ("Rack Id"=w207:u8, "State"=w193:string)
            n66 = Equal?(x=w198, y="Master Sample") -> (x = y?=w196:bool)
            n67 = Select(t="MS", s=w196, f=w193) -> (s? t:f=w194:string)
            n68 = Bundle By Name(cluster=w204, "Output Cluster.Part Info.Rack ID"=w207, "Output Cluster.Part Info.Part Name"=w198, "Output Cluster.Part Info.MeasurementIDsArray"=w206, "Output Cluster.Part Info.Measurement Names Array"=w205, "Output Cluster.Part Info.Spec Values Array"=w201, "State"=w194) -> (w203:T3)
            n69 = flat-sequence {
              tunnel: [w212] -> w200
              tunnel: w199 -> [w212]
              frame #0 {
                n70 = Wait (ms)(milliseconds to wait=u32 100) -> ()  [unwired: 1 out]
              }
            }
            n71 = call <vilib>:"Add State(s) to Queue__JKI_lib_State_Machine.vi"("State(s) in Front (\"\")"="GetCameraDetails" ("State(s) in Front (\"\")"), "State(s) in (\"\")"=w210) -> ("States Out"=w209:string)  [unwired: 13 in]
          }
          event User Event {
            # "All part info"
            n72 = event-data() -> ("AllPartInfo"=w217:T9)  [unwired: 1 in]
            n73 = Unbundle By Name(w221) -> ("Output Cluster"=w219:T5)
            n74 = Bundle By Name(cluster=w219, "AllPartInfo"=w217) -> (w218:T5)
            n75 = call "Output_RC.vi"("Rack Controller in"=w220, "Output Cluster"=w218, "Receiver Name"="Parent", "State"="AllPartInfo", "error in (no error)"=w215) -> ("error out"=w214:errorcluster)  [unwired: 10 in]
            n76 = call <vilib>:"Add State(s) to Queue__JKI_lib_State_Machine.vi"("State(s) in (\"\")"=w223) -> ("States Out"=w222:string)  [unwired: 14 in]
          }
          event User Event {
            # "Camera info"
            n77 = event-data() -> ("Camera Names"=w225:string[], "Number of Active Cameras"=w226:u8)  [unwired: 1 in]
            n78 = Bundle By Name(cluster=w228, "Output Cluster.Part Info.Camera Names Array"=w225, "Part Details.Number Of Cameras"=w226) -> (w227:T3)
            n79 = call <vilib>:"Add State(s) to Queue__JKI_lib_State_Machine.vi"("State(s) in Front (\"\")"="SendInitialization\nInitBuffer" ("State(s) in Front (\"\")"), "State(s) in (\"\")"=w232) -> ("States Out"=w231:string)  [unwired: 13 in]
          }
          event User Event {
            # "Result data"
            n80 = event-data() -> ("Measurement Values Array"=w260:dbl[], "Images Array"=w259:T1[], "Result PF"=w248:bool, "Control PF Array"=w258:bool[], "Specification PF Array"=w257:bool[], "Specification Fail?"=w256:bool)  [unwired: 1 in, 2 out]
            n81 = Unbundle By Name(w240) -> ("State"=w238:string, "CountDetails"=w239:T15)
            n82 = call "UpdatingCount_RC.vi"("error in"=w247, "CountDetails"=w239, "Pass/Fail"=w248) -> ("error out"=w243:errorcluster, "Reel Counter Result"=w246:T13, "Total Cluster Result"=w245:T16, "CountDetailsOut"=w244:T15)  [unwired: 5 in]
            n83 = Bundle By Name(cluster=w240, "CountDetails"=w244) -> (w241:T3)
            n84 = Unbundle By Name(w241) -> ("Output Cluster"=w242:T5)
            n85 = Equal?(x=w238, y="MS") -> (x = y?=w236:bool)
            n86 = in-place {
              in-place-border: w260 -> [w265]
              in-place-border: w259 -> [w266]
              in-place-border: w248 -> [w267]
              in-place-border: w258 -> [w270]
              in-place-border: w257 -> [w271]
              in-place-border: w246 -> [w269]
              in-place-border: w256 -> [w272]
              in-place-border: w245 -> [w268]
              n87 = in-place-cluster #2(w241) -> ("Rack Id"=w264:u8, "Reel Number"=w263:u64)
              n88 = in-place-cluster #3(w242) -> ()  [unwired: 11 out]
              n89 = in-place-cluster #3("Result Cluster.RackID"=w264, "Result Cluster.ReelNumber"=w263, "Result Cluster.MeasurementValuesArray"=w265, "Result Cluster.ImagesArray"=w266, "Result Cluster.ResultPF"=w267, "Result Cluster.ProductionCountDetails"=w268, "Result Cluster.ReelCountDetails"=w269, "Result Cluster.ControlPFArray"=w270, "Result Cluster.SpecificationPFArray"=w271, "Result Cluster.SpecificationFail"=w272, "Result Cluster.Status"="") -> (w249:T5)
              n90 = in-place-cluster #2("Rack Id"=w264, "Reel Number"=w263) -> (w251:T3)
            }
            n91 = Select(t="", s=w236, f="AnalyzeResult" ("State(s) in Front (\"\")")) -> (s? t:f=w234:string)
            n92 = call <vilib>:"Add State(s) to Queue__JKI_lib_State_Machine.vi"("State(s) in Front (\"\")"=w234, "State(s) in (\"\")"=w261) -> ("States Out"=w262:string)  [unwired: 13 in]
            n93 = call "Output_RC.vi"("Rack Controller in"=w254, "Output Cluster"=w249, "Receiver Name"="Parent", "State"="Result to Parent", "error in (no error)"=w243) -> ("error out"=w255:errorcluster)  [unwired: 10 in]
            n94 = Bundle By Name(cluster=w251, "Output Cluster"=w249) -> (w250:T3)
          }
          event User Event {
            # "Pause event from tracking loop"
            n95 = event-data() -> ("RackID"=w285:u8, "MeasurementValuesArray"=w284:dbl[], "ImagesArray"=w283:T1[], "ResultPF"=w282:bool, "ProductionCountDetails"=w281:T17, "ReelCountDetails"=w280:T18, "ControlPFArray"=w279:bool[], "SpecificationPFArray"=w278:bool[], "SpecificationFail"=w277:bool, "ReelNumber"=w276:u64, "Status"=w275:string)  [unwired: 1 in]
            n96 = Unbundle By Name(w286) -> ("Output Cluster"=w288:T5)
            n97 = in-place {
              in-place-border: w285 -> [w306]
              in-place-border: w284 -> [w305]
              in-place-border: w283 -> [w304]
              in-place-border: w282 -> [w303]
              in-place-border: w281 -> [w302]
              in-place-border: w280 -> [w301]
              in-place-border: w279 -> [w300]
              in-place-border: w278 -> [w299]
              in-place-border: w277 -> [w298]
              in-place-border: w276 -> [w297]
              in-place-border: w275 -> [w296]
              n98 = in-place-cluster #4(w288) -> ()  [unwired: 11 out]
              n99 = in-place-cluster #4("Result Cluster.RackID"=w306, "Result Cluster.MeasurementValuesArray"=w305, "Result Cluster.ImagesArray"=w304, "Result Cluster.ResultPF"=w303, "Result Cluster.ProductionCountDetails"=w302, "Result Cluster.ReelCountDetails"=w301, "Result Cluster.ControlPFArray"=w300, "Result Cluster.SpecificationPFArray"=w299, "Result Cluster.SpecificationFail"=w298, "Result Cluster.ReelNumber"=w297, "Result Cluster.Status"=w296) -> (w287:T5)
            }
            n100 = call <vilib>:"Add State(s) to Queue__JKI_lib_State_Machine.vi"("State(s) in Front (\"\")"="Pause" ("State(s) in Front (\"\")"), "State(s) in (\"\")"=w294) -> ("States Out"=w295:string)  [unwired: 13 in]
            n101 = call "Output_RC.vi"("Rack Controller in"=w291, "Output Cluster"=w287, "Receiver Name"="Parent", "State"="Result to Parent", "error in (no error)"=w293) -> ("error out"=w292:errorcluster)  [unwired: 10 in]
          }
          event Panel Close? {
            # "Discard the event because we'll close the front panel ourselves in Macro: Exit"
            # "Close Panel button (pressed) Event\n(this executes Macro: Exit to terminate the VI)"
            # "Panel close"
            n102 = event-data() -> ()  [unwired: 1 in, 1 out]
            n103 = call <vilib>:"Add State(s) to Queue__JKI_lib_State_Machine.vi"("State(s) in Front (\"\")"="Macro: Exit", "State(s) in (\"\")"=w313) -> ("States Out"=w312:string)  [unwired: 13 in]
            n104 = event-data("Discard?"=TRUE) -> ()  [unwired: 1 in, 1 out]
          }
        }
      }
      frame "---------- Core ----------" {
        # "Do not put any code in this frame.\n(it is a separator no-op)"
        n105 = call <vilib>:"Add State(s) to Queue__JKI_lib_State_Machine.vi"("State(s) in (\"\")"=w318) -> ("States Out"=w317:string)  [unwired: 14 in]
      }
      frame Default {
        w329 = 42 items=["No error", "Argument error", "Memory is full", "Out of zone", "End of file", "File already open", "Generic file I/O error", "File not found", "File permission error", "Disk is full", "Duplicate path", "Too many files open", "System feature not enabled", "Resource file not found", "Cannot add resource", "Resource not found", "Image not found", "Image memory error", "Pen does not exist", "Config type invalid", "Config token not found", "Config parse error", "Config memory error", "Bad external code format", "Bad external code offset", "External code not present", "Null window", "Destroy window error", "Null menu", "Print aborted", "Bad print record", "Print driver error", "Windows error during printing", "Memory error during printing", "Print dialog error", "Generic print error", "Invalid device refnum", "Device not found", "Device parameter error", "Device unit error", "Cannot open device", "Device call aborted", "Generic error", "Cancelled by user", "Object ID too low", "Object ID too high", "Object not in heap", "Unknown heap", "Unknown object (invalid DefProc)", "Unknown object (DefProc not in table)", "Message out of range", "Invalid (null) method", "Unknown message", "Manager call not supported", "Bad address", "Network operation in progress", "Network operation timed out", "Connection is busy", "Network attribute not supported", "Network error", "Address in use", "System out of memory", "Connection aborted", "Connection refused", "Not connected", "Already connected", "Connection closed", "Initialization error (interapplication manager)", "Bad occurrence", "Wait on unbound occurrence handler", "Occurrence queue overflow", "Datalog type conflict", "Unused", "Unrecognized type (interapplication manager)", "Memory corrupt", "Failed to make temporary DLL", "Old CIN version", "Drag socket not found", "Failed to load drop-object", "Failed to register OLE object", "Failed to release OLE object", "Format specifier type mismatch", "Unknown format specifier", "Too few format specifiers", "Too many format specifiers", "Scan failed", "Newer CIN version", "Error converting to variant", "Runtime menu error", "Password tampered", "Variant attribute not found", "Incompatible variant data type", "Event data is not available", "Event Store is not present", "Occurrence is not found", "Event Queue is not created", "Event info is not available", "Refnum passed is NULL", "Error retrieving Class GUID", "Error retrieving CoClass GUID", "Error retrieving TypeLib GUID.", "Bad built application magic bytes.", "Specific driver is different from the specific driver associated with the Logical Name.", "There is no session opened to the class driver.", "Max Error", "MAX - Error with config objects", "MAX - Error loading configuration", "MAX - Group not supported"]
        # "Current State"
        # "Do not delete, rename, or modify this frame.\n(this is used to capture unhandled states and typos)"
        # "Handle mistyped state name (developer tool)"
        n106 = Format Into String(format string="Software Exception: Unhandled State \"%s\"." ("message"), error in=w325, w322) -> (resulting string=w328:string, error out=w327:errorcluster)  [unwired: 1 in]
        n107 = call <vilib>:"Error Cluster From Error Code.vi"("show call chain? (False)"=TRUE, "error in (no error)"=w327, "error message (\"\")"=w328, "error code (0)"=w329) -> ("error out"=w326:errorcluster)  [unwired: 5 in]
        n108 = call <vilib>:"Add State(s) to Queue__JKI_lib_State_Machine.vi"("State(s) in (\"\")"=w324) -> ("States Out"=w323:string)  [unwired: 14 in]
      }
      frame "Initialize Core Data" {
        # "Do not delete, rename, or modify this frame.\n(this is used to determine panel behavior on exit)"
        # "originally closed?"
        # "exe?"
        # "If panel starts closed or is an EXE, then close it when we exit"
        n109 = property class="VI"() -> ("Front Panel.Open"=w339:bool)  [unwired: 2 in, 2 out]
        n110 = property class="App"() -> ("App.Kind"=w338:T10)  [unwired: 2 in, 2 out]
        n111 = control-ref of="Current VI Reference"() -> (w333:refnum<vi>)
        n112 = Not(x=w339) -> (.not. x?=w336:bool)
        n113 = Equal?(x=w338, y=T10."Run Time System" ("Application:Kind")) -> (x = y?=w335:bool)
        n114 = Or(x=w336, y=w335) -> (x .or. y?=w331:bool)
        n115 = Bundle By Name(cluster=w334, "Core.Current VI Reference"=w333, "Core.Close Panel on Exit?"=w331) -> (w341:T3)
        n116 = call <vilib>:"Add State(s) to Queue__JKI_lib_State_Machine.vi"("State(s) in (\"\")"=w343) -> ("States Out"=w342:string)  [unwired: 14 in]
      }
      frame "Error Handler" {
        # "Handle any errors here.\nYou can also output any states to clean-up after errors occur"
        # "Clear error"
        n117 = Unbundle By Name(w349) -> ("Output Cluster"=w348:T5)
        n118 = Bundle By Name(cluster=w348, "Error Message"="RackControllerError_0xF500") -> (w346:T5)
        n119 = call "Output_RC.vi"("Rack Controller in"=w350, "Output Cluster"=w346, "Receiver Name"="Parent", "State"="Error Message") -> ()  [unwired: 11 in, 1 out]
        n120 = call <vilib>:"Add State(s) to Queue__JKI_lib_State_Machine.vi"("State(s) in Front (\"\")"="/* Post Error States", "State(s) in (\"\")"=w354) -> ("States Out"=w353:string)  [unwired: 13 in]
      }
      frame "Exit" {
        # "Do not put any code in this frame.\n(No errors that occur here will be handled.)"
        n121 = call <vilib>:"Add State(s) to Queue__JKI_lib_State_Machine.vi"("State(s) in (\"\")"=w360) -> ("States Out"=w359:string)  [unwired: 14 in]
      }
      frame "---------- Data ----------" {
        # "Do not put any code in this frame.\n(It is a separator no-op. You can make a copy of this frame to create a new Data frame)"
        n122 = call <vilib>:"Add State(s) to Queue__JKI_lib_State_Machine.vi"("State(s) in (\"\")"=w365) -> ("States Out"=w364:string)  [unwired: 14 in]
      }
      frame "Data: Initialize" {
        w366 = T15 {"Total Cluster Values"={"Total Fail"=0, "Total Pass"=0, "Total Count"=0}, "Reel Counter Cluster"={"Reel Fail"=0, "Reel Pass"=0, "Reel Count"=0}}  # CountDetails
        w367 = FALSE  # Update
        w378 = T4 {"Name"="", "Unload Position Counts"={"Fail"=0, "Reel End"=0, "Production End"=0}, "Number Of Cameras"=0, "Measurement Details Array"=[], "Reel Count"=0, "Total Count"=0}  # Part Details
        w379 = T19 {"HardwareEmulated"=TRUE, "DefectTrackingEnable"=TRUE, "PauseOnReelCountFinish"=TRUE, "StopOnTotalCountFinish"=TRUE}  # System Info_RC
        w370 = T5 {"Acknowledgement"={"Actor Enqueuer"=refnum, "VI Reference"=refnum, "VI Name"=""}, "Rack ID"=0, "Clear"=FALSE, "Light Camera Info"={"Light Camera Name"="", " State"=""}, "Camera Optics Diagnostics Result"={"LightCameraName"="", "DiagnosedImage"=refnum, "DustPercentage"=0.0, "Result"=TRUE}, "Receiver Enqueuer"={"Actor Enqueuer"=refnum, "VI Name"=""}, "Error Message"="", "Part Details"={"Part Name"="", "Total Count"=0, "Reel Count"=0}, "Result Cluster"={"RackID"=0, "MeasurementValuesArray "=[], "ImagesArray"=[], "ResultPF"=FALSE, "ProductionCountDetails"={"TotalFail"=0, "TotalPass"=0, "TotalCount"=0}, "ReelCountDetails"={"ReelFail"=0, "ReelPass"=0, "ReelCount"=0}, "ControlPFArray"=[], "SpecificationPFArray"=[], "SpecificationFail"=FALSE, "ReelNumber"=0, "Status"=""}, "Part Info"={"Part Name"="", "Rack ID"=0, "MeasurementIDsArray"=[], "Measurement Names Array"=[], "Spec Values Array"=[], "Camera Names Array"=[], "Total count"=0, "Reel count"=0}, "AllPartInfo"=[{"PartName"="", "NumberOfRacks"=0, "MeasurementIDsArray"=[], "MeasurementNamesArray"=[], "SpecValuesArray"=[]}], "ImagesAndCount"={"Image Array"=[], "ImageCount"=0}}  # Output Cluster
        w380 = u64 0  # Reel Number
        w384 = ""  # State
        w385 = TRUE  # Send Run to CC?
        w387 = TRUE  # First Call?
        w388 = 0  # Ack
        w389 = T20 {"Current VI Reference"=refnum, "Close Panel on Exit?"=FALSE}  # Core
        # "Initialize the shift-register data, here.\n(data names are defined by what you wire into the bundle function)"
        n123 = Unbundle By Name(w376) -> ("RC Parameters Path"=w375:path, "RC Override file path"=w374:path)
        n124 = Decimal String To Number(string=w386) -> (offset past number=w369:i32, number=w377:i32)  [unwired: 2 in]
        n125 = call "JSON reading_RC.vi"("error in"=w373, "Override file path"=w374, "Default file path"=w375) -> ("error out"=w372:errorcluster, "Output Merged Cluster"=w371:variant)  [unwired: 7 in]
        n126 = Bundle By Name(cluster=w370, "Part Info.Rack ID"=w369) -> (w368:T5)
        n127 = Bundle By Name(cluster=T3 {"Timeout"=0, "Core"={"Current VI Reference"=refnum, "Close Panel on Exit?"=FALSE}, "Rack Id"=0, "Part Details"={"Name"="", "Unload Position Counts"={"Fail"=0, "Reel End"=0, "Production End"=0}, "Number Of Cameras"=0, "Measurement Details Array"=[], "Reel Count"=0, "Total Count"=0}, "Ack"=0, "First Call?"=FALSE, "Send Run to CC?"=FALSE, "State"="", "Reel Number"=0, "Output Cluster"={"Acknowledgement"={"Actor Enqueuer"=refnum, "VI Reference"=refnum, "VI Name"=""}, "Rack ID"=0, "Clear"=FALSE, "Light Camera Info"={"Light Camera Name"="", " State"=""}, "Camera Optics Diagnostics Result"={"LightCameraName"="", "DiagnosedImage"=refnum, "DustPercentage"=0.0, "Result"=TRUE}, "Receiver Enqueuer"={"Actor Enqueuer"=refnum, "VI Name"=""}, "Error Message"="", "Part Details"={"Part Name"="", "Total Count"=0, "Reel Count"=0}, "Result Cluster"={"RackID"=0, "MeasurementValuesArray "=[], "ImagesArray"=[], "ResultPF"=FALSE, "ProductionCountDetails"={"TotalFail"=0, "TotalPass"=0, "TotalCount"=0}, "ReelCountDetails"={"ReelFail"=0, "ReelPass"=0, "ReelCount"=0}, "ControlPFArray"=[], "SpecificationPFArray"=[], "SpecificationFail"=FALSE, "ReelNumber"=0, "Status"=""}, "Part Info"={"Part Name"="", "Rack ID"=0, "MeasurementIDsArray"=[], "Measurement Names Array"=[], "Spec Values Array"=[], "Camera Names Array"=[], "Total count"=0, "Reel count"=0}, "AllPartInfo"=[{"PartName"="", "NumberOfRacks"=0, "MeasurementIDsArray"=[], "MeasurementNamesArray"=[], "SpecValuesArray"=[]}], "ImagesAndCount"={"Image Array"=[], "ImageCount"=0}}, "System Info_RC"={"HardwareEmulated"=TRUE, "DefectTrackingEnable"=TRUE, "PauseOnReelCountFinish"=TRUE, "StopOnTotalCountFinish"=TRUE}, "Rack based Parameters"=variant, "Update"=FALSE, "CountDetails"={"Total Cluster Values"={"Total Fail"=0, "Total Pass"=0, "Total Count"=0}, "Reel Counter Cluster"={"Reel Fail"=0, "Reel Pass"=0, "Reel Count"=0}}}, "Timeout"=-1, "Core"=w389, "Rack Id"=w377, "Part Details"=w378, "Ack"=w388, "First Call?"=w387, "Send Run to CC?"=w385, "State"=w384, "Reel Number"=w380, "Output Cluster"=w368, "System Info_RC"=w379, "Rack based Parameters"=w371, "Update"=w367, "CountDetails"=w366) -> (w383:T3)
        n128 = call <vilib>:"Add State(s) to Queue__JKI_lib_State_Machine.vi"("State(s) in (\"\")"=w391) -> ("States Out"=w390:string)  [unwired: 14 in]
      }
      frame "Data: Cleanup" {
        # "Cleanup any data and references, here.\n(this is called automatically, by the Macro: Exit)"
        n129 = Unregister For Events(event registration refnum=w397, error in=w396) -> (error out=w395:errorcluster)
        n130 = call "Destroy User Events_RC.vi"("error in (no error)"=w395, "Rack Controller in"=w393) -> ("error out"=w394:errorcluster)  [unwired: 9 in]
        n131 = Unbundle By Name(w398) -> ("Core.Current VI Reference"=w392:refnum<vi>)
        n132 = Close Reference(reference=w392, error in (no error)=w394) -> (error out=w399:errorcluster)
        n133 = call <vilib>:"Add State(s) to Queue__JKI_lib_State_Machine.vi"("State(s) in (\"\")"=w401) -> ("States Out"=w400:string)  [unwired: 14 in]
      }
      frame "---------- UI ----------" {
        # "Do not put any code in this frame.\n(It is a separator no-op. You can make a copy of this frame to create a new UI frame)"
        n134 = call <vilib>:"Add State(s) to Queue__JKI_lib_State_Machine.vi"("State(s) in (\"\")"=w406) -> ("States Out"=w405:string)  [unwired: 14 in]
      }
      frame "UI: Initialize" {
        # "Initialize the User Interface, here.\n(this is called automatically, by the Macro: Init)"
        n135 = call <vilib>:"Add State(s) to Queue__JKI_lib_State_Machine.vi"("State(s) in (\"\")"=w411) -> ("States Out"=w410:string)  [unwired: 14 in]
      }
      frame "UI: Front Panel State" {
        # "Argument"
        # "Set Front Panel Open or Closed\n(Usage: \"UI: Front Panel State >> Open|Close\")"
        n136 = Unbundle By Name(w415) -> ("Core.Current VI Reference"=w413:refnum<vi>)
        n137 = case shown="\"Open\", Default" w412 {
          tunnel: w417 -> [w423 w436]
          tunnel: [w425 w437] -> w416
          tunnel: w413 -> [w424 w434]
          frame "Open", Default {
            n138 = property class="VI"(reference=w424, error in=w423) -> (reference out=w421:refnum<vi>, error out=w422:errorcluster, "Front Panel.Open"=w420:bool)
            n139 = case shown="False" w420 {
              tunnel: [w428 w431] -> w425
              tunnel: w422 -> [w427 w431]
              tunnel: w421 -> [w426 _]
              frame False {
                n140 = invoke class="VI" method="FP.Open"(reference=w426, error in=w427, "Activate"=TRUE, "State"=T11."Standard") -> (error out=w428:errorcluster)  [unwired: 1 in, 4 out]
              }
              frame True {
              }
            }
          }
          frame "Close" {
            n141 = property class="VI"(reference=w434, error in=w436) -> (reference out=w433:refnum<vi>, error out=w435:errorcluster, "Front Panel.Open"=w432:bool)
            n142 = case shown="True" w432 {
              tunnel: [w438 w441] -> w437
              tunnel: w435 -> [w438 w440]
              tunnel: w433 -> [_ w439]
              frame False {
              }
              frame True {
                n143 = invoke class="VI" method="FP.Close"(reference=w439, error in=w440) -> (error out=w441:errorcluster)  [unwired: 1 in, 2 out]
              }
            }
          }
        }
        n144 = call <vilib>:"Add State(s) to Queue__JKI_lib_State_Machine.vi"("State(s) in (\"\")"=w419) -> ("States Out"=w418:string)  [unwired: 14 in]
      }
      frame "---------- Macro ----------" {
        # "Do not put any code in this frame.\n(It is a separator no-op. You can make a copy of this frame to create a new Macro frame)"
        n145 = call <vilib>:"Add State(s) to Queue__JKI_lib_State_Machine.vi"("State(s) in (\"\")"=w446) -> ("States Out"=w445:string)  [unwired: 14 in]
      }
      frame "Macro: Initialize" {
        # "Acknowledgement is sent to Inspection Statemachine.\nWait for Rack Id from SM"
        # "Initialization Macro\n(This is called once, when the VI starts)"
        n146 = call <vilib>:"Add State(s) to Queue__JKI_lib_State_Machine.vi"("State(s) in Front (\"\")"="Acknowledgement", "State(s) in (\"\")"=w452) -> ("States Out"=w451:string)  [unwired: 13 in]
      }
      frame "Macro: Exit" {
        # "Exit Macro\n(This is called once, when the VI exits)"
        n147 = Unbundle By Name(w461) -> ("Core.Close Panel on Exit?"=w460:bool)
        n148 = Select(t="UI: Front Panel State >> Close", s=w460, f="") -> (s? t:f=w454:string)
        n149 = call <vilib>:"Add State(s) to Queue__JKI_lib_State_Machine.vi"("State(s) in Front (\"\")"=w454, "State(s) at Back (\"\")"="Data: Cleanup\nExit") -> ("States Out"=w455:string)  [unwired: 13 in]
        n150 = call <vilib>:"Add State(s) to Queue__JKI_lib_State_Machine.vi"("State(s) in Front (\"\")"=w455, "State(s) in (\"\")"=w464) -> ("States Out"=w463:string)  [unwired: 13 in]
      }
      frame "---------- Launch ----------" {
        # "Template Separator\n(You can make a copy of, or modify, this frame)"
        n151 = call <vilib>:"Add State(s) to Queue__JKI_lib_State_Machine.vi"("State(s) in (\"\")"=w469) -> ("States Out"=w468:string)  [unwired: 14 in]
      }
      frame "Acknowledgement" {
        # "Do not put any code in this frame.\n(it is a separator no-op)"
        n152 = call <vilib>:"Read Self Enqueuer.vi"("Actor"=w480) -> ("Self Enqueuer"=w479:refnum<class "Message Enqueuer.lvclass">)  [unwired: 10 in]
        n153 = control-ref of="This VI"() -> (w478:refnum<vi>)
        n154 = Bundle By Name(cluster=T5 {"Acknowledgement"={"Actor Enqueuer"=refnum, "VI Reference"=refnum, "VI Name"=""}, "Rack ID"=0, "Clear"=FALSE, "Light Camera Info"={"Light Camera Name"="", " State"=""}, "Camera Optics Diagnostics Result"={"LightCameraName"="", "DiagnosedImage"=refnum, "DustPercentage"=0.0, "Result"=TRUE}, "Receiver Enqueuer"={"Actor Enqueuer"=refnum, "VI Name"=""}, "Error Message"="", "Part Details"={"Part Name"="", "Total Count"=0, "Reel Count"=0}, "Result Cluster"={"RackID"=0, "MeasurementValuesArray "=[], "ImagesArray"=[], "ResultPF"=FALSE, "ProductionCountDetails"={"TotalFail"=0, "TotalPass"=0, "TotalCount"=0}, "ReelCountDetails"={"ReelFail"=0, "ReelPass"=0, "ReelCount"=0}, "ControlPFArray"=[], "SpecificationPFArray"=[], "SpecificationFail"=FALSE, "ReelNumber"=0, "Status"=""}, "Part Info"={"Part Name"="", "Rack ID"=0, "MeasurementIDsArray"=[], "Measurement Names Array"=[], "Spec Values Array"=[], "Camera Names Array"=[], "Total count"=0, "Reel count"=0}, "AllPartInfo"=[{"PartName"="", "NumberOfRacks"=0, "MeasurementIDsArray"=[], "MeasurementNamesArray"=[], "SpecValuesArray"=[]}], "ImagesAndCount"={"Image Array"=[], "ImageCount"=0}} ("Output Cluster"), "Acknowledgement.Actor Enqueuer"=w479, "Acknowledgement.VI Reference"=w478) -> (w477:T5)
        n155 = call "Output_RC.vi"("Rack Controller in"=w480, "Output Cluster"=w477, "Receiver Name"="Parent", "State"="Acknowledgement", "error in (no error)"=w482) -> ("error out"=w481:errorcluster)  [unwired: 10 in]
        n156 = Bundle By Name(cluster=w473, "Timeout"=-1) -> (w472:T3)
        n157 = call <vilib>:"Add State(s) to Queue__JKI_lib_State_Machine.vi"("State(s) in Front (\"\")"="Wait" ("State(s) in Front (\"\")"), "State(s) in (\"\")"=w484) -> ("States Out"=w483:string)  [unwired: 13 in]
      }
      frame "LaunchActors" {
        w485 = refnum<class "Camera Controller.lvclass"> refnum  # Camera Controller.lvclass
        w486 = refnum<class "Algorithm.lvclass"> refnum  # Algorithm.lvclass
        # "Camera Controller and Algorithm Actors \nare launched waits for Acknowledgement"
        n158 = call <vilib>:"Launch Nested Actor.vi"("error in (no error)"=w490, "Nested Actor"=w485, "Caller Actor in"=w487) -> ("error out"=w489:errorcluster)  [unwired: 6 in, 2 out]
        n159 = call <vilib>:"Launch Nested Actor.vi"("error in (no error)"=w489, "Nested Actor"=w486, "Caller Actor in"=w487) -> ("error out"=w488:errorcluster)  [unwired: 6 in, 2 out]
        n160 = call <vilib>:"Add State(s) to Queue__JKI_lib_State_Machine.vi"("State(s) in Front (\"\")"="Wait" ("State(s) in Front (\"\")"), "State(s) in (\"\")"=w494) -> ("States Out"=w493:string)  [unwired: 13 in]
      }
      frame "SendChildIds" {
        n161 = Unbundle By Name(w506) -> ("Output Cluster"=w504:T5, "Rack Id"=w503:u8)
        n162 = Bundle By Name(cluster=w504, "Rack ID"=w503) -> (w497:T5)
        n163 = call "Output_RC.vi"("Rack Controller in"=w498, "Output Cluster"=w497, "Receiver Name"="ZenCAM", "State"="Rack ID to ZenCAM", "error in (no error)"=w505) -> ("error out"=w496:errorcluster)  [unwired: 10 in]
        n164 = call "Output_RC.vi"("Rack Controller in"=w498, "Output Cluster"=w497, "Receiver Name"="Algorithm", "State"="Rack ID to Algorithm", "error in (no error)"=w496) -> ("error out"=w495:errorcluster)  [unwired: 10 in]
        n165 = call <vilib>:"Add State(s) to Queue__JKI_lib_State_Machine.vi"("State(s) in (\"\")"=w508) -> ("States Out"=w507:string)  [unwired: 14 in]
      }
      frame "SendEnqueuer" {
        # "Algo enqueuer to be sent to CC"
        n166 = Unbundle By Name(w512) -> ("Algorithm Actor's Enqueuer"=w511:refnum<class "Message Enqueuer.lvclass">)
        n167 = Unbundle By Name(w515) -> ("Output Cluster"=w510:T5)
        n168 = Bundle By Name(cluster=w510, "Receiver Enqueuer.Actor Enqueuer"=w511) -> (w509:T5)
        n169 = call "Output_RC.vi"("Rack Controller in"=w512, "Output Cluster"=w509, "Receiver Name"="ZenCAM", "State"="Algo Enqueuer to ZenCAM", "error in (no error)"=w517) -> ("error out"=w516:errorcluster)  [unwired: 10 in]
        n170 = call <vilib>:"Add State(s) to Queue__JKI_lib_State_Machine.vi"("State(s) in (\"\")"=w518) -> ("States Out"=w519:string)  [unwired: 14 in]
      }
      frame "Select" {
        n171 = call <vilib>:"Add State(s) to Queue__JKI_lib_State_Machine.vi"("State(s) in Front (\"\")"="Wait" ("State(s) in Front (\"\")"), "State(s) in (\"\")"=w525) -> ("States Out"=w524:string)  [unwired: 13 in]
      }
      frame "GetCameraDetails" {
        n172 = Unbundle By Name(w530) -> ("Output Cluster"=w528:T5)
        n173 = call "Output_RC.vi"("Rack Controller in"=w529, "Output Cluster"=w528, "Receiver Name"="ZenCAM", "State"="GetCameraDetails", "error in (no error)"=w532) -> ("error out"=w531:errorcluster)  [unwired: 10 in]
        n174 = call <vilib>:"Add State(s) to Queue__JKI_lib_State_Machine.vi"("State(s) in (\"\")"=w534) -> ("States Out"=w533:string)  [unwired: 14 in]
      }
      frame "SendInitialization" {
        n175 = Unbundle By Name(w538) -> ("Output Cluster"=w535:T5)
        n176 = call "Output_RC.vi"("Rack Controller in"=w541, "Output Cluster"=w535, "Receiver Name"="Parent", "State"="Initialization", "error in (no error)"=w540) -> ("error out"=w539:errorcluster)  [unwired: 10 in]
        n177 = call <vilib>:"Add State(s) to Queue__JKI_lib_State_Machine.vi"("State(s) in (\"\")"=w543) -> ("States Out"=w542:string)  [unwired: 14 in]
      }
      frame "PartSelected" {
        n178 = in-place {
          in-place-border: w548 -> [w562]
          in-place-border: [w561] -> w547
          n179 = in-place-cluster #5(w545) -> ("Part Details"=w560:T4, "Rack based Parameters"=w557:variant, "Rack Id"=w556:u8)  [unwired: 2 out]
          n180 = Unbundle By Name(w560) -> ("Name"=w559:string)
          n181 = call "Read Part Details_RC.vi"("Part Details in"=w560, "error in (no error)"=w562, "Rack ID"=w556, "Part Name"=w559, "Output Merged Cluster"=w557) -> ("error out"=w561:errorcluster, "Part Details out"=w558:T4)  [unwired: 5 in]
          n182 = in-place-cluster #5("Part Details"=w558, "Rack based Parameters"=w557, "Rack Id"=w556, "Send Run to CC?"=TRUE, "State"="PartSelected" ("Previous State")) -> (w546:T3)
        }
        n183 = Unbundle By Name(w545) -> ("Output Cluster"=w544:T5)
        n184 = case shown="Error" w547 {
          selector: w547 -> [w563 _]
          tunnel: [w563 w565] -> w551
          tunnel: w550 -> [_ w568]
          tunnel: w544 -> [_ w571]
          frame No Error {
          }
          frame Error {
            # "JSON reading Error"
            n185 = Bundle By Name(cluster=w571, "Error Message"="RackControllerError_0xF501") -> (w569:T5)
            n186 = call "Output_RC.vi"("Rack Controller in"=w568, "Output Cluster"=w569, "Receiver Name"="Parent", "State"="Error Message", "error in (no error)"=errorcluster {"status"=FALSE, "code"=0, "source"=""}) -> ("error out"=w565:errorcluster)  [unwired: 10 in]
          }
        }
        n187 = call <vilib>:"Add State(s) to Queue__JKI_lib_State_Machine.vi"("State(s) in Front (\"\")"="SendPartDetails" ("State(s) in Front (\"\")"), "State(s) in (\"\")"=w553) -> ("States Out"=w552:string)  [unwired: 13 in]
      }
      frame "SendPartDetails" {
        # "code modified_RC\nchanged \"OutputCluster\" out to \n\"PartDetails\""
        n188 = Unbundle By Name(w585) -> ("Output Cluster"=w576:T5, "Part Details.Name"=w575:string, "Part Details.Total Count"=w574:u64, "Part Details.Reel Count"=w573:u64)
        n189 = Bundle By Name(cluster=w576, "Part Details.Part Name"=w575, "Part Details.Total Count"=w574, "Part Details.Reel Count"=w573) -> (w572:T5)
        n190 = call "Output_RC.vi"("Rack Controller in"=w584, "Output Cluster"=w572, "Receiver Name"="ZenCAM", "State"="Part Details to ZenCAM", "error in (no error)"=w578) -> ("error out"=w579:errorcluster)  [unwired: 10 in]
        n191 = call "Output_RC.vi"("Rack Controller in"=w584, "Output Cluster"=w572, "Receiver Name"="Algorithm", "State"="Part Details to Algo", "error in (no error)"=w579) -> ("error out"=w577:errorcluster)  [unwired: 10 in]
        n192 = call <vilib>:"Add State(s) to Queue__JKI_lib_State_Machine.vi"("State(s) in (\"\")"=w587) -> ("States Out"=w586:string)  [unwired: 14 in]
      }
      frame "Update" {
        n193 = Unbundle By Name(w606) -> ("Part Details"=w592:T4, "Part Details.Name"=w588:string, "Rack Id"=w593:u8, "Output Cluster"=w598:T5)
        n194 = call "Output_RC.vi"("Rack Controller in"=w599, "Output Cluster"=w598, "Receiver Name"="Algorithm", "State"="Update to Algorithm", "error in (no error)"=w600) -> ("error out"=w597:errorcluster)  [unwired: 10 in]
        n195 = Unbundle By Name(w599) -> ("RC Parameters Path"=w605:path, "RC Override file path"=w604:path)
        n196 = call "JSON reading_RC.vi"("error in"=w597, "Override file path"=w604, "Default file path"=w605) -> ("error out"=w596:errorcluster, "Output Merged Cluster"=w595:variant)  [unwired: 7 in]
        n197 = Equal?(x=w588, y="") -> (x = y?=w589:bool)
        n198 = case shown="False" w589 {
          tunnel: w596 -> [w616 w617]
          tunnel: w595 -> [w615 _]
          tunnel: [w614 w618] -> w594
          tunnel: w593 -> [w613 _]
          tunnel: w588 -> [w610 _]
          tunnel: w592 -> [w612 w618]
          tunnel: [w611 w617] -> w591
          frame False {
            n199 = call "Read Part Details_RC.vi"("Part Details in"=w612, "error in (no error)"=w616, "Rack ID"=w613, "Part Name"=w610, "Output Merged Cluster"=w615) -> ("error out"=w611:errorcluster, "Part Details out"=w614:T4)  [unwired: 5 in]
          }
          frame True {
          }
        }
        n200 = call <vilib>:"Add State(s) to Queue__JKI_lib_State_Machine.vi"("State(s) in (\"\")"=w609) -> ("States Out"=w608:string)  [unwired: 14 in]
        n201 = Bundle By Name(cluster=w606, "Part Details"=w594, "State"="Update" ("Previous State")) -> (w607:T3)
      }
      frame "InitBuffer" {
        # "This State is not called if \nDefect Tracking feature is disabled"
        n202 = Unbundle By Name(w624) -> ("Part Details.Unload Position Counts"=w621:T21, "Part Details.Number Of Cameras"=w620:u8)
        n203 = Bundle By Name(cluster=T12 {"Unload Position Counts"={"Fail"=0, "ReelEnd"=0, "ProductionEnd"=0}, "Number of Cameras"=0} ("event data"), "Unload Position Counts"=w621, "Number of Cameras"=w620) -> (w619:T12)
        n204 = Unbundle By Name(w623) -> ("Init to Tracking Loop"=w627:refnum<user-event>)
        n205 = Generate User Event(user event=w627, event data cluster=w619, error in=w626) -> (error out=w625:errorcluster)  [unwired: 1 in, 1 out]
        n206 = call <vilib>:"Add State(s) to Queue__JKI_lib_State_Machine.vi"("State(s) in (\"\")"=w629) -> ("States Out"=w628:string)  [unwired: 14 in]
      }
      frame "Run" {
        n207 = Unbundle By Name(w632) -> ("System Info_RC.HardwareEmulated"=w630:bool, "Send Run to CC?"=w636:bool, "Output Cluster"=w633:T5)
        n208 = case shown="True" w636 {
          tunnel: w637 -> [w650 w656]
          tunnel: [w650 w655] -> w635
          tunnel: w634 -> [_ w654]
          tunnel: w633 -> [_ w653]
          frame False {
          }
          frame True {
            n209 = call "Output_RC.vi"("Rack Controller in"=w654, "Output Cluster"=w653, "Receiver Name"="ZenCAM", "State"="Run to ZenCAM", "error in (no error)"=w656) -> ("error out"=w655:errorcluster)  [unwired: 10 in]
          }
        }
        n210 = in-place {
          in-place-border: w630 -> [w646]
          n211 = in-place-cluster #6(w632) -> ("State"=w645:string)  [unwired: 1 out]
          n212 = Equal?(x=w645, y="MS") -> (x = y?=w643:bool)
          n213 = Select(t=TRUE ("Send Run to CC?"), s=w646, f=FALSE ("Send Run to CC?")) -> (s? t:f=w647:bool)
          n214 = Select(t="MS", s=w643, f="Run" ("Previous State")) -> (s? t:f=w640:string)
          n215 = in-place-cluster #6("Send Run to CC?"=w647, "State"=w640) -> (w631:T3)
        }
        n216 = call <vilib>:"Add State(s) to Queue__JKI_lib_State_Machine.vi"("State(s) in (\"\")"=w639) -> ("States Out"=w638:string)  [unwired: 14 in]
      }
      frame "AnalyzeResult" {
        w684 = T22 {"Result Cluster"={"Rack ID"=0, "Measurement Values Array "=[], "Images Array"=[], "Result PF"=FALSE, "Production Count Details"={"Total Fail"=0, "Total Pass"=0, "Total Count"=0}, "Reel Count Details"={"Reel Fail"=0, "Reel Pass"=0, "Reel Count"=0}, "Control PF Array"=[], "Specification PF Array"=[], "Specification Fail?"=FALSE, "Reel Number"=0, "Status"=""}, "Pause on Fail?"=FALSE, "Total Count Finish?"=FALSE, "Reel Count Finish?"=FALSE}  # event data
        n217 = Unbundle By Name(w666) -> ("CountDetails.Reel Counter Cluster"=w663:T13, "CountDetails.Total Cluster Values"=w660:T16)
        n218 = Unbundle By Name(w666) -> ("System Info_RC.StopOnTotalCountFinish"=w675:bool, "Part Details.Total Count"=w673:u64, "Output Cluster.Result Cluster.ProductionCountDetails.TotalCount"=w674:u64)
        n219 = Unbundle By Name(w666) -> ("System Info_RC.PauseOnReelCountFinish"=w680:bool, "Part Details.Reel Count"=w679:u64, "Output Cluster.Result Cluster.ReelCountDetails.ReelCount"=w678:u64)
        n220 = Unbundle By Name(w666) -> ("Output Cluster.Result Cluster"=w668:T8)
        n221 = Equal?(x=w679, y=w678) -> (x = y?=w664:bool)
        n222 = Equal?(x=w673, y=w674) -> (x = y?=w659:bool)
        n223 = Select(t=w664, s=w680, f=FALSE) -> (s? t:f=w672:bool)
        n224 = Select(t=w659, s=w675, f=FALSE) -> (s? t:f=w665:bool)
        n225 = Select(t=T13 {"Reel Fail"=0, "Reel Pass"=0, "Reel Count"=0}, s=w664, f=w663) -> (s? t:f=w657:T13)
        n226 = Select(t=T13 {"Reel Fail"=0, "Reel Pass"=0, "Reel Count"=0}, s=w659, f=w660) -> (s? t:f=w658:T16)
        n227 = call "Measurement-wise MN logic.vi"("cluster"=w666) -> ("Pause On Fail"=w667:bool, "Measurement Details Array"=w671:T23)  [unwired: 9 in]
        n228 = call <vilib>:"Add State(s) to Queue__JKI_lib_State_Machine.vi"("State(s) in (\"\")"=w687) -> ("States Out"=w686:string)  [unwired: 14 in]
        n229 = Bundle By Name(cluster=w666, "Part Details.Measurement Details Array"=w671, "CountDetails.Reel Counter Cluster"=w657, "CountDetails.Total Cluster Values"=w658) -> (w670:T3)
        n230 = Bundle By Name(cluster=w684, "Result Cluster"=w668, "Pause on Fail?"=w667, "Reel Count Finish?"=w672, "Total Count Finish?"=w665) -> (w683:T22)
        n231 = Unbundle By Name(w682) -> ("Result to Track"=w685:refnum<user-event>)
        n232 = Generate User Event(user event=w685, event data cluster=w683, error in=w669) -> (error out=w681:errorcluster)  [unwired: 1 in, 1 out]
      }
      frame "Pause" {
        n233 = Unbundle By Name(w689) -> ("State Message_RC"=w697:refnum<user-event>, "IgnoredFailCountDetails_RC"=w688:refnum<user-event>)
        n234 = Unbundle By Name(w692) -> ("Send Run to CC?"=w699:bool, "Output Cluster"=w691:T5)
        n235 = case shown="True" w699 {
          tunnel: w704 -> [w708 w712]
          tunnel: [w708 w711] -> w693
          tunnel: w691 -> [_ w709]
          tunnel: w689 -> [_ w710]
          frame False {
          }
          frame True {
            n236 = call "Output_RC.vi"("Rack Controller in"=w710, "Output Cluster"=w709, "Receiver Name"="ZenCAM", "State"="Pause to ZenCAM", "error in (no error)"=w712) -> ("error out"=w711:errorcluster)  [unwired: 10 in]
          }
        }
        n237 = register-events(w697, w688) -> (reference out=w703:refnum<event-registration>)  [unwired: 2 in, 1 out]
        n238 = Bundle By Name(cluster=w692, "First Call?"=TRUE, "State"="Pause" ("Previous State")) -> (w695:T3)
        n239 = while {
          tunnel: w703 -> [w724]
          tunnel: [w723] -> w702
          shift-right: [w715] -> w701
          shift-left: w693 -> [w721]
          tunnel: w698 -> [w720]
          tunnel: w689 -> [w719]
          tunnel: [w716] -> w690
          shift-right: [w717] -> w694
          shift-left: w695 -> [w718]
          stop <- w722 stop-if-true
          n240 = event shown="[1] <IgnoredFailCountDetails_RC>: User Event" {
            selector: w724 -> [_ _]
            dyn-events: [_ _] -> w723
            timeout: _ -> [_ _]
            tunnel: [w727 FALSE] -> w722
            tunnel: w721 -> [w730 w784]
            tunnel: w720 -> [w732 _]
            tunnel: w719 -> [w729 _]
            tunnel: w718 -> [w726 w779]
            tunnel: [w725 w774] -> w717
            tunnel: [w731 ""] -> w716
            tunnel: [w728 w784] -> w715
            event User Event {
              n241 = event-data() -> ("State Message_RC"=w733:string)  [unwired: 1 in]
              n242 = case shown="\"Update\"" w733 {
                selector: w733 -> [w738 w744 _ _]
                tunnel: w732 -> [w739 w745 _ _]
                tunnel: [w738 w744 "" ""] -> w731
                tunnel: w730 -> [w737 w742 w749 w757]
                tunnel: w729 -> [_ _ _ w763]
                tunnel: [w736 w743 w749 w768] -> w728
                tunnel: [TRUE TRUE TRUE FALSE] -> w727
                tunnel: w726 -> [w734 w740 w746 w761]
                tunnel: [w734 w740 w746 w762] -> w725
                frame "SoftwareExit" {
                  # "Name of software\nexit is \"SoftwareExit\"\nand not \"Software Exit\""
                  # "code modified_RC"
                  n243 = Flush Event Queue(0:w739, 3:w737) -> (11:w736:errorcluster)  [unwired: 4 in, 2 out]
                }
                frame "Stop" {
                  n244 = Flush Event Queue(0:w745, 3:w742) -> (11:w743:errorcluster)  [unwired: 4 in, 2 out]
                }
                frame "Run", Default {
                  # "Run case has been converted to the default case"
                  # "code modified_RC"
                }
                frame "Update" {
                  n245 = Unbundle By Name(w761) -> ("Output Cluster"=w764:T5, "Rack Id"=w751:u8, "Part Details.Name"=w753:string, "Part Details"=w750:T4)
                  n246 = Unbundle By Name(w763) -> ("RC Parameters Path"=w759:path, "RC Override file path"=w758:path)
                  n247 = call "JSON reading_RC.vi"("error in"=w757, "Override file path"=w758, "Default file path"=w759) -> ("error out"=w756:errorcluster, "Output Merged Cluster"=w754:variant)  [unwired: 7 in]
                  n248 = call "Read Part Details_RC.vi"("Part Details in"=w750, "error in (no error)"=w756, "Rack ID"=w751, "Part Name"=w753, "Output Merged Cluster"=w754) -> ("error out"=w755:errorcluster, "Part Details out"=w752:T4)  [unwired: 5 in]
                  n249 = call "Output_RC.vi"("Rack Controller in"=w763, "Output Cluster"=w764, "Receiver Name"="Algorithm", "State"="Update to Algorithm", "error in (no error)"=w757) -> ("error out"=w769:errorcluster)  [unwired: 10 in]
                  n250 = Bundle By Name(cluster=w761, "Part Details"=w752) -> (w762:T3)
                  n251 = Merge Errors(w769, w755) -> (w768:errorcluster)
                }
              }
            }
            event User Event {
              n252 = event-data() -> ("TotalCount"=w781:u64, "ReelCount"=w780:u64)  [unwired: 1 in]
              n253 = Unbundle By Name(w779) -> ("CountDetails.Total Cluster Values.Total Pass"=w782:u64, "CountDetails.Total Cluster Values.Total Fail"=w773:u64, "CountDetails.Reel Counter Cluster.Reel Pass"=w772:u64, "CountDetails.Reel Counter Cluster.Reel Fail"=w771:u64)
              n254 = Add(x=w782, y=w781) -> (x+y=w778:u64)
              n255 = Subtract(x=w773, y=w781) -> (x-y=w777:u64)
              n256 = Add(x=w772, y=w780) -> (x+y=w776:u64)
              n257 = Subtract(x=w771, y=w780) -> (x-y=w775:u64)
              n258 = Bundle By Name(cluster=w779, "CountDetails.Total Cluster Values.Total Pass"=w778, "CountDetails.Total Cluster Values.Total Fail"=w777, "CountDetails.Reel Counter Cluster.Reel Pass"=w776, "CountDetails.Reel Counter Cluster.Reel Fail"=w775) -> (w774:T3)
            }
          }
        }
        n259 = call <vilib>:"Add State(s) to Queue__JKI_lib_State_Machine.vi"("State(s) in Front (\"\")"=w690, "State(s) in (\"\")"=w707) -> ("States Out"=w706:string)  [unwired: 13 in]
        n260 = Unregister For Events(event registration refnum=w702, error in=w701) -> (error out=w700:errorcluster)
      }
      frame "Stop" {
        w785 = T15 {"Total Cluster Values"={"Total Fail"=0, "Total Pass"=0, "Total Count"=0}, "Reel Counter Cluster"={"Reel Fail"=0, "Reel Pass"=0, "Reel Count"=0}}  # CountDetails
        # "Reinitialize variables"
        n261 = Flush Event Queue(0:w798, 3:w787) -> (11:w786:errorcluster)  [unwired: 4 in, 2 out]
        n262 = Unbundle By Name(w789) -> ("Output Cluster"=w788:T5)
        n263 = call "Output_RC.vi"("Rack Controller in"=w790, "Output Cluster"=w788, "Receiver Name"="ZenCAM", "State"="Stop to ZenCAM", "error in (no error)"=w786) -> ("error out"=w796:errorcluster)  [unwired: 10 in]
        n264 = call "Output_RC.vi"("Rack Controller in"=w790, "Output Cluster"=w788, "Receiver Name"="Algorithm", "State"="Stop to Algorithm", "error in (no error)"=w796) -> ("error out"=w795:errorcluster)  [unwired: 10 in]
        n265 = Bundle By Name(cluster=w789, "State"="Stop" ("Previous State"), "CountDetails"=w785) -> (w799:T3)
        n266 = call <vilib>:"Add State(s) to Queue__JKI_lib_State_Machine.vi"("State(s) in Front (\"\")"="Wait" ("State(s) in Front (\"\")"), "State(s) in (\"\")"=w802) -> ("States Out"=w801:string)  [unwired: 13 in]
      }
      frame "SensorDiagnostics" {
        n267 = Unbundle By Name(w807) -> ("Output Cluster"=w806:T5)
        n268 = call "Output_RC.vi"("Rack Controller in"=w809, "Output Cluster"=w806, "Receiver Name"="ZenCAM", "State"="Sensor Diagnostics", "error in (no error)"=w803) -> ("error out"=w808:errorcluster)  [unwired: 10 in]
        n269 = call <vilib>:"Add State(s) to Queue__JKI_lib_State_Machine.vi"("State(s) in Front (\"\")"="Wait" ("State(s) in Front (\"\")"), "State(s) in (\"\")"=w812) -> ("States Out"=w811:string)  [unwired: 13 in]
      }
      frame "StopSensorDiagnostics" {
        n270 = Unbundle By Name(w817) -> ("Output Cluster"=w816:T5)
        n271 = call "Output_RC.vi"("Rack Controller in"=w819, "Output Cluster"=w816, "Receiver Name"="ZenCAM", "State"="Stop Sensor Diagnostics", "error in (no error)"=w813) -> ("error out"=w818:errorcluster)  [unwired: 10 in]
        n272 = call <vilib>:"Add State(s) to Queue__JKI_lib_State_Machine.vi"("State(s) in Front (\"\")"="Wait" ("State(s) in Front (\"\")"), "State(s) in (\"\")"=w822) -> ("States Out"=w821:string)  [unwired: 13 in]
      }
      frame "SoftwareExit" {
        # "Do not put any code in this frame.\n(it is a separator no-op)"
        n273 = Unbundle By Name(w825) -> ("Stop Tracking loop"=w827:refnum<user-event>, "Algorithm Actor's Enqueuer"=w829:refnum<class "Message Enqueuer.lvclass">, "Camera Controller Actor's Enqueuer"=w831:refnum<class "Message Enqueuer.lvclass">)
        n274 = call <vilib>:"Send Normal Stop.vi"("error in (no error)"=w824, "Message Enqueuer"=w831) -> ("error out"=w830:errorcluster)  [unwired: 9 in]
        n275 = call <vilib>:"Send Normal Stop.vi"("error in (no error)"=w830, "Message Enqueuer"=w829) -> ("error out"=w828:errorcluster)  [unwired: 9 in]
        n276 = Generate User Event(user event=w827, event data cluster=TRUE ("event data"), error in=w828) -> (error out=w823:errorcluster)  [unwired: 1 in, 1 out]
        n277 = call <vilib>:"Add State(s) to Queue__JKI_lib_State_Machine.vi"("State(s) in Front (\"\")"="Macro: Exit" ("State(s) in Front (\"\")"), "State(s) in (\"\")"=w835) -> ("States Out"=w834:string)  [unwired: 13 in]
      }
    }
  }
  n278 = while {
    shift-right: [w840] -> _
    shift-left: w7 -> [w841]
    tunnel: w6 -> [w839]
    shift-right: [w837] -> w3
    shift-left: w4 -> [w836]
    tunnel: "Rack Controller in" -> [w838]
    stop <- w842 stop-if-true
    # "Tracking loop"
    n279 = event shown="[3] <Stop Tracking loop>: User Event" {
      selector: w839 -> [_ _ _ w1023]
      dyn-events: _ -> [_ _ _ _]
      timeout: _ -> [_ _ _ _]
      tunnel: [_ _ _ w1021] -> w842
      tunnel: w841 -> [w845 w936 w953 w1031]
      tunnel: [w844 w937 w952 w1031] -> w840
      tunnel: w838 -> [w847 _ _ w1022]
      tunnel: w836 -> [w849 w926 w954 w1024]
      tunnel: [w848 w925 w960 w1019] -> w837
      event User Event {
        n280 = event-data() -> ("Global Count Value Change_RC"=w843:u64)  [unwired: 1 in]
        n281 = Unbundle By Name(w847) -> ("Pause event from Tracking loop"=w846:refnum<user-event>)
        n282 = in-place {
          in-place-border: w849 -> [w891]
          in-place-border: [w880] -> w848
          in-place-border: w846 -> [w870]
          in-place-border: w843 -> [w867]
          w871 = usereventprio."high priority" ("priority (normal)")
          # "Check for Total finish"
          # "Check for Reel finish"
          # "Check for fail"
          n283 = in-place-cluster #7(w845) -> ("Buffer"=w873:T25, "Result"=w872:T22, "Check Pos 3"=w869:u32, "Check Pos 2"=w860:u32, "Check Pos 1"=w857:u32)  [unwired: 1 out]
          n284 = Delete From Array(array=w873, index=w869) -> (array with subset deleted=w879:T25)  [unwired: 1 in, 1 out]
          n285 = To Long Integer(number=w869) -> (32bit integer=w866:i32)
          n286 = Insert Into Array(array=w879, index=0, new element=w872) -> (w863:T25)
          n287 = Index Array(array=w863, index=w866) -> (element=w874:T22)
          n288 = Unbundle By Name(w874) -> ("Pause on Fail?"=w894:bool, "Result Cluster"=w875:T26)
          n289 = Bundle By Name(cluster=w875, "Status"="Fail" ("Result data")) -> (w890:T26)
          n290 = Equal?(x=w894, y=TRUE) -> (x = y?=w892:bool)
          n291 = case shown="True" w892 {
            tunnel: w891 -> [w909 w913]
            tunnel: w890 -> [_ w911]
            tunnel: [w909 w914] -> w887
            tunnel: w870 -> [_ w912]
            tunnel: w871 -> [_ w910]
            frame False {
            }
            frame True {
              # "on fail"
              n292 = Generate User Event(priority (normal)=w910, user event=w912, event data cluster=w911, error in=w913) -> (error out=w914:errorcluster)  [unwired: 1 out]
            }
          }
          n293 = To Long Integer(number=w857) -> (32bit integer=w865:i32)
          n294 = Index Array(array=w863, index=w865) -> (element=w886:T22)
          n295 = Unbundle By Name(w886) -> ("Total Count Finish?"=w856:bool, "Result Cluster"=w859:T26)
          n296 = Bundle By Name(cluster=w859, "Status"="TotalFinish" ("Result data")) -> (w889:T26)
          n297 = Equal?(x=w856, y=TRUE) -> (x = y?=w888:bool)
          n298 = case shown="True" w888 {
            tunnel: w887 -> [w903 w906]
            tunnel: w889 -> [_ w907]
            tunnel: [w903 w908] -> w882
            tunnel: w870 -> [_ w904]
            tunnel: w871 -> [_ w905]
            frame False {
            }
            frame True {
              # "on reel finish"
              n299 = Generate User Event(priority (normal)=w905, user event=w904, event data cluster=w907, error in=w906) -> (error out=w908:errorcluster)  [unwired: 1 out]
            }
          }
          n300 = To Long Integer(number=w860) -> (32bit integer=w864:i32)
          n301 = Index Array(array=w863, index=w864) -> (element=w881:T22)
          n302 = Select(t="y", s=w856, f="n") -> (s? t:f=w853:string)
          n303 = Unbundle By Name(w881) -> ("Reel Count Finish?"=w885:bool, "Result Cluster"=w858:T26)
          n304 = case shown="\"n\", Default" w853 {
            tunnel: [TRUE FALSE] -> w851
            frame "n", Default {
            }
            frame "y" {
            }
          }
          n305 = Bundle By Name(cluster=w858, "Status"="ReelFinish" ("Result data")) -> (w883:T26)
          n306 = Equal?(x=w885, y=TRUE) -> (x = y?=w852:bool)
          n307 = And(x=w851, y=w852) -> (x .and. y?=w850:bool)
          n308 = case shown="True" w850 {
            tunnel: w882 -> [w897 w900]
            tunnel: w883 -> [_ w901]
            tunnel: [w897 w902] -> w880
            tunnel: w870 -> [_ w899]
            tunnel: w871 -> [_ w898]
            frame False {
            }
            frame True {
              # "on total finish"
              n309 = Generate User Event(priority (normal)=w898, user event=w899, event data cluster=w901, error in=w900) -> (error out=w902:errorcluster)  [unwired: 1 out]
            }
          }
          n310 = in-place-cluster #7("Global Count"=w867, "Buffer"=w863, "Result"=T22 {"Result Cluster"={"Rack ID"=0, "Measurement Values Array "=[], "Images Array"=[], "Result PF"=FALSE, "Production Count Details"={"Total Fail"=0, "Total Pass"=0, "Total Count"=0}, "Reel Count Details"={"Reel Fail"=0, "Reel Pass"=0, "Reel Count"=0}, "Control PF Array"=[], "Specification PF Array"=[], "Specification Fail?"=FALSE, "Reel Number"=0, "Status"=""}, "Pause on Fail?"=FALSE, "Total Count Finish?"=FALSE, "Reel Count Finish?"=FALSE}, "Check Pos 3"=w869, "Check Pos 2"=w860, "Check Pos 1"=w857) -> (w844:T2)
        }
      }
      event User Event {
        w921 = 1
        w932 = T22 {"Result Cluster"={"Rack ID"=0, "Measurement Values Array "=[], "Images Array"=[], "Result PF"=TRUE, "Production Count Details"={"Total Fail"=0, "Total Pass"=0, "Total Count"=0}, "Reel Count Details"={"Reel Fail"=0, "Reel Pass"=0, "Reel Count"=0}, "Control PF Array"=[], "Specification PF Array"=[], "Specification Fail?"=FALSE, "Reel Number"=0, "Status"=""}, "Pause on Fail?"=FALSE, "Total Count Finish?"=FALSE, "Reel Count Finish?"=FALSE}  # Result
        w933 = u32 0  # Initial value
        # "Initializing Image buffer with the \nmaximum reject position as the row \nsize and the number of cameras \nused as column size. The image \nname in the buffer is given as\n \" Image <row index> <column index>."
        # "To initialize buffer size with the maximum reject\n position value and update the check position 1, 2 \nand 3 with the least reject position value, middle \nreject position value and maximum reject position\n value respectively."
        n311 = event-data() -> ("Unload Position Counts.Fail"=w918:u32, "Unload Position Counts.ReelEnd"=w919:u32, "Unload Position Counts.ProductionEnd"=w920:u32, "Number of Cameras"=w929:u8)  [unwired: 1 in]
        n312 = Build Array(w918, w919, w920) -> (w928:u32[])
        n313 = Equal To 0?(x=w918) -> (x = 0?=w924:bool)
        n314 = Array Max & Min(array=w928) -> (max value=w927:u32)  [unwired: 3 out]
        n315 = Equal To 0?(x=w919) -> (x = 0?=w923:bool)
        n316 = Equal To 0?(x=w920) -> (x = 0?=w922:bool)
        n317 = Select(t=w921, s=w924, f=w918) -> (s? t:f=w915:u32)
        n318 = for {
          N: w915 -> [_]
          tunnel: [w941] -> w930 mode=indexing
          tunnel: w929 -> [w940]
          tunnel: w926 -> [w939]
          tunnel: [w938] -> w925
          i -> [w942]
          n319 = for {
            N: w940 -> [_]
            tunnel: w942 -> [w950]
            tunnel: [w945] -> w941 mode=indexing
            tunnel: w939 -> [w944]
            tunnel: [w943] -> w938
            i -> [w951]
            n320 = Number To Decimal String(number=w950) -> (decimal integer string=w949:string)  [unwired: 1 in]
            n321 = Number To Decimal String(number=w951) -> (decimal integer string=w948:string)  [unwired: 1 in]
            n322 = Concatenate Strings("Image", w949, w948) -> (w946:string)
            n323 = call "IMAQ Create"("Image Name"=w946, "error in (no error)"=w944) -> ("New Image"=w945:T1, "error out"=w943:errorcluster)  [unwired: 3 in]
          }
        }
        n324 = Select(t=w921, s=w923, f=w919) -> (s? t:f=w917:u32)
        n325 = To Long Integer(number=w927) -> (32bit integer=w935:i32)
        n326 = Select(t=w921, s=w922, f=w920) -> (s? t:f=w916:u32)
        n327 = Initialize Array(T22 {"Result Cluster"={"Rack ID"=0, "Measurement Values Array "=[], "Images Array"=[], "Result PF"=TRUE, "Production Count Details"={"Total Fail"=0, "Total Pass"=0, "Total Count"=0}, "Reel Count Details"={"Reel Fail"=0, "Reel Pass"=0, "Reel Count"=0}, "Control PF Array"=[], "Specification PF Array"=[], "Specification Fail?"=FALSE, "Reel Number"=0, "Status"=""}, "Pause on Fail?"=FALSE, "Total Count Finish?"=FALSE, "Reel Count Finish?"=FALSE} ("output cluster"), w935) -> (w934:T25)
        n328 = Bundle By Name(cluster=w936, "Buffer Size"=w927, "Global Count"=w933, "Result Count"=w933, "Buffer"=w934, "Result"=w932, "Check Pos 3"=w915, "Check Pos 2"=w917, "Check Pos 1"=w916, "Image buffer"=w930) -> (w937:T2)
      }
      event User Event {
        n329 = event-data() -> ("Result Cluster.Production Count Details.Total Count"=w955:u64, "Result Cluster"=w959:T26, "Pause on Fail?"=w958:bool, "Total Count Finish?"=w957:bool, "Reel Count Finish?"=w956:bool)  [unwired: 1 in]
        n330 = in-place {
          in-place-border: [w982] -> w960
          in-place-border: w959 -> [w980]
          in-place-border: w958 -> [w979]
          in-place-border: w957 -> [w978]
          in-place-border: w956 -> [w977]
          in-place-border: w955 -> [w976]
          in-place-border: w954 -> [w974]
          w981 = T22 {"Result Cluster"={"Rack ID"=0, "Measurement Values Array "=[], "Images Array"=[], "Result PF"=TRUE, "Production Count Details"={"Total Fail"=0, "Total Pass"=0, "Total Count"=0}, "Reel Count Details"={"Reel Fail"=0, "Reel Pass"=0, "Reel Count"=0}, "Control PF Array"=[], "Specification PF Array"=[], "Specification Fail?"=FALSE, "Reel Number"=0, "Status"=""}, "Pause on Fail?"=FALSE, "Total Count Finish?"=FALSE, "Reel Count Finish?"=FALSE}  # Result to Track
          # "The row at which the image is \nto be inserted is indexed out \nand the columns accept \nthe corresponding images \nby for loop auto indexing."
          n331 = in-place-cluster #8(w953) -> ("Buffer"=w970:T25, "Result Count"=w969:u32, "Global Count"=w961:u32, "Buffer Size"=w966:u32, "Image buffer"=w968:T1[][])
          n332 = Bundle By Name(cluster=w981, "Result Cluster"=w980, "Pause on Fail?"=w979, "Total Count Finish?"=w978, "Reel Count Finish?"=w977) -> (w983:T22)
          n333 = To Unsigned Long Integer(number=w976) -> (unsigned 32bit integer=w975:u32)
          n334 = Subtract(x=w961, y=w975) -> (x-y=w973:u32)
          n335 = Quotient & Remainder(x=w975, y=w966) -> (x-y*floor(x/y)=w963:u32)  [unwired: 1 out]
          n336 = Greater?(x=w973, y=w966) -> (0:w984:bool)
          n337 = To Long Integer(number=w963) -> (32bit integer=w962:i32)
          n338 = case shown="False" w984 {
            tunnel: w969 -> [w999 w1017]
            tunnel: [w995 w1017] -> w971
            tunnel: w973 -> [w996 _]
            tunnel: w970 -> [w997 w1016]
            tunnel: w983 -> [w987 _]
            tunnel: [w998 w1016] -> w972
            tunnel: [w990 w1015] -> w982
            tunnel: w974 -> [w991 w1015]
            tunnel: w968 -> [w989 w1014]
            tunnel: [w985 w1014] -> w964
            tunnel: w961 -> [w994 w1013]
            tunnel: [w994 w1013] -> w967
            tunnel: [w993 w1012] -> w965
            tunnel: w966 -> [w993 w1012]
            tunnel: w962 -> [w988 _]
            frame False {
              # "To update the result value to the buffer at corresponding positions"
              n339 = Unbundle By Name(w987) -> ("Result Cluster.Images Array"=w986:T1[])
              n340 = for {
                shift-right: [w1005] -> w990
                shift-left: w991 -> [w1006]
                tunnel: w988 -> [w1003]
                tunnel: w986 -> [w1001] mode=indexing
                shift-right: [w1000] -> w985
                shift-left: w989 -> [w1004]
                i -> [w1002]
                n341 = in-place {
                  in-place-border: w1006 -> [w1011]
                  in-place-border: [w1010] -> w1005
                  in-place-border: w1001 -> [w1008]
                  n342 = in-place-array #9(w1004, w1003, w1002) -> (w1009:T1)
                  n343 = call "IMAQ Copy"("error in (no error)"=w1011, "Image Dst"=w1009, "Image Src"=w1008) -> ("error out"=w1010:errorcluster, "Image Dst Out"=w1007:T1)  [unwired: 3 in]
                  n344 = in-place-array #9(w1007) -> (w1000:T1[][])  [unwired: 2 out]
                }
              }
              n345 = To Long Integer(number=w996) -> (32bit integer=w992:i32)
              n346 = Replace Array Subset(array=w997, new element=w987, index=w992) -> (w998:T25)
              n347 = Increment(x=w999) -> (x+1=w995:u32)
            }
            frame True {
              # "Result is obtained after terminal crosses reject position"
            }
          }
          n348 = in-place-cluster #8("Buffer"=w972, "Result Count"=w971, "Global Count"=w967, "Buffer Size"=w965, "Image buffer"=w964) -> (w952:T2)
        }
      }
      event User Event {
        n349 = event-data() -> ("Stop_Track"=w1021:bool)  [unwired: 1 in]
        n350 = Unbundle By Name(w1022) -> ("Current Trigger Count_RC"=w1018:refnum<user-event>, "Result to Track"=w1027:refnum<user-event>, "State Message_RC"=w1026:refnum<user-event>, "Rack ID_RC"=w1025:refnum<user-event>)
        n351 = Unregister For Events(event registration refnum=w1023, error in=w1024) -> (error out=w1030:errorcluster)
        n352 = Destroy User Event(user event=w1027, error in=w1030) -> (error out=w1029:errorcluster)
        n353 = Destroy User Event(user event=w1026, error in=w1029) -> (error out=w1028:errorcluster)
        n354 = Destroy User Event(user event=w1025, error in=w1028) -> (error out=w1020:errorcluster)
        n355 = Destroy User Event(user event=w1018, error in=w1020) -> (error out=w1019:errorcluster)
      }
    }
  }
  n356 = Merge Errors(w31, w28, w3) -> (→"error out":errorcluster)
